vi "Dashboard Main.vi"() -> ()   [LabVIEW 2015]
uses:
  Robot Code/Autonomous Mode.ctl
  <vilib>/Utility/miscctls.llb/LVPointTypeDef.ctl
  <vilib>/Utility/miscctls.llb/LVPositionTypeDef.ctl
  <vilib>/Utility/miscctls.llb/LVRectTypeDef.ctl
  <vilib>/Utility/miscctls.llb/LVRowAndColumnTypeDef.ctl
  <vilib>/event_ctls.llb/eventvkey.ctl
  Operator-Interface-Control-Board.git/trunk/LabVIEW/PWM_Output_TypeDef.ctl
  Operator-Interface-Control-Board.git/trunk/LabVIEW/LED_Output_TypeDef.ctl
  <vilib>/Rock Robotics/Network Tables/NT Read Numeric Array.vi
  <vilib>/Rock Robotics/Network Tables/NT Read Boolean Array.vi
  <vilib>/Rock Robotics/Network Tables/NT Write Boolean Array.vi
  <vilib>/Rock Robotics/Network Tables/NT Write Numeric Array.vi
  <vilib>/Rock Robotics/Network Tables/NT Read Boolean.vi
  <vilib>/Rock Robotics/WPI/Dashboard/WPI_DashboardLogging Global.vi
  <vilib>/vision/driver/NI_Vision_Acquisition_Software.lvlib
panel:
  in  "TCP":refnum<k5>
  out "Image Message":string="Timeout in Camera Communications"
  in  "Dashboard Tab":T1(tab)
  out "Right Drive Speed":dbl(knob) scale=20.0..-20.0
  out "Left Drive Speed":dbl(knob) scale=-20.0..20.0
  out "Robot Direction":dbl(knob) scale=0.0..360.0
  out "Arm Lock State":bool
  out "Distance":string
  out "Front Distance":dbl(slide) scale=0.0..25.0 scale format="%#_g ft"
  out "Arm Mode":string="Disconnected"
  out "Arm Information":cluster{dbl, dbl}(knob)={90.0, 90.0} scale=90.0..220.0 scale format="%d°"
  out "Autonomous Selection":T2
  out "Air Presure":dbl(slide) scale=0.0..150.0 scale format="%#_1f"
  out "Control Board Connection":bool
  out "Network Table Connection":bool
  out "MotorChart R":cluster{"Numeric":dbl, "Numeric":dbl}(graph)
  out "MotorChart L":T3(graph)
  out "MotorSliders R":cluster{"MotorSlide1":dbl, "MotorSlide2":dbl} {"MotorSlide2" scale=-1.0..1.0 scale format="%#_2e"; "MotorSlide1" scale=-1.0..1.0 scale format="%#_2e"}
  out "MotorSliders L":T4 {"MotorSlide4 2" scale=0.0..14.0 scale format="%#_2e"; "MotorSlide2" scale=-1.0..1.0 scale format="%#_2e"; "MotorSlide1" scale=-1.0..1.0 scale format="%#_2e"}
  out "JS1 Z":dbl(slide) scale=-1.0..1.0 scale format="%#_2e"
  out "JS1 Graph":cluster{"X":dbl, "Y":dbl}[](graph)
  out "JS1 Buttons":T5
  out "JS2 Z":dbl(slide) scale=-1.0..1.0 scale format="%#_2e"
  out "JS2 Graph":cluster{"X":dbl, "Y":dbl}[](graph)
  out "JS2 Buttons":T5
  out "Mode":T6(ring)=enum."Auto Disabled"
  in  "DB Camera Config":bool
  out "fps":dbl format="%#.1g"
  out "Mbps":dbl format="%#.1g"
  out "Mbps LED":bool
  in  "Test Slider":dbl(slide) scale=0.0..100.0 scale format="%#_3g"
  in  "On/Off":bool caption="Solenoid"
  in  "Test Name":u16(ring) items=["Select the test to run..."]
  in  "Test Tree":string(tree)
  in  "Motor":cluster{"Value":dbl, "Enable":bool} {"Value" scale=-1.0..1.0 scale format="%#_3g"}
  out "Progress":T7 {"Test Progress" scale=0.0..100.0}
  in  "Rev/Fwd":cluster{"Forward":bool, "Reverse":bool}
  in  "Test Ring":u16(ring) items=["Monochrome", "Color"]
  out "Cmd Status":string
  in  "Execute Command":bool
  in  "Command Params":string[][](table)
  in  "Command Selection":i32(listbox)
  in  "CheckList":i32(listbox)
  out "Tree":string(tree)
  out "Camera Image":T8(plugin-control)
  # "Current"
  # "Set"
  # "Left"
  # "Front"
  # "Right"
  # "Battery"
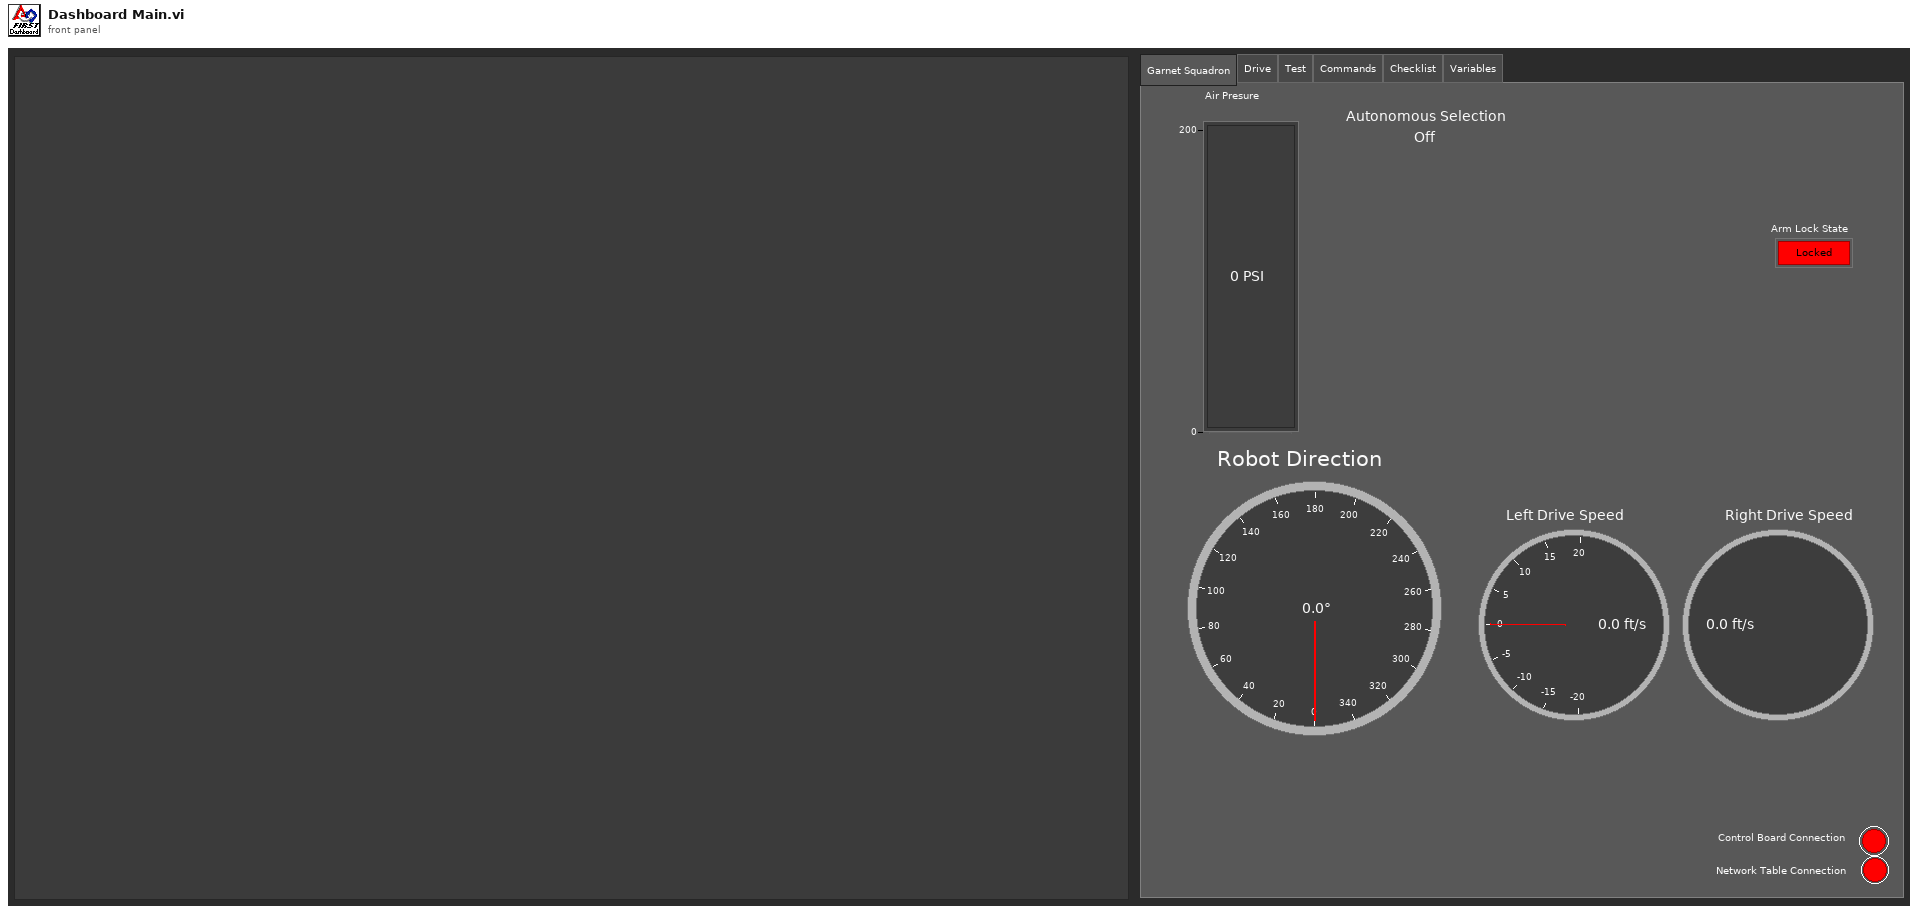
[diagram p1: front panel]
types:
  T1 = enum32{"Garnet Squadron", "Drive", "Test", "Commands", "Checklist", "Variables"}
  T2 = typedef "Autonomous Mode.ctl" = enum16{"Off", "Cross Defense", "Shoot A/B", "Shoot C/D", "Shoot E"}
  T3 = cluster{"Numeric":dbl, "Numeric":dbl, "Battery V":dbl}
  T4 = cluster{"MotorSlide1":dbl, "MotorSlide2":dbl, "MotorSlide4 2":dbl}
  T5 = cluster{bool, bool, bool, bool, bool, bool, bool, bool, bool, bool, bool, bool}
  T6 = enum8{"Tele-Op Disabled", "Tele-Op Enabled", "Auto Disabled", "Auto Enabled", "Test Disabled", "Test Enabled", "Disconnected", "No Code", "E-Stop"}
  T7 = cluster{"Test Progress":u8, "Test Progress Text":string}
  T8 = typedef "IMAQ Image.ctl" = refnum<image>
  T9 = enum32{"Invalid", "Default", "Floating", "Floating/Auto-Hide", "Modal"}
  T10 = typedef "LVRectTypeDef.ctl" = cluster{"Left":i16, "Top":i16, "Right":i16, "Bottom":i16}
  T11 = typedef "LVPositionTypeDef.ctl" = cluster{"Left":i32, "Top":i32}
  T12 = typedef "LVPointTypeDef.ctl" = cluster{"Horizontal":i16, "Vertical":i16}
  T13 = cluster{"IDs":cluster{"RPC field ID":u16, "Unique ID":u16}, "String":string}
  T14 = enum32{"Drive", "Basic", "Custom", "Test", "Checklist", "Variables"}
  T15 = typedef "Image Type" = u32
  T16 = cluster{"Desired Font (Application)":enum16{"User-specified Font", "Application Font", "System Font", "Dialog Font"}, "[User-specified Font]":cluster{"Font Name":string, "Size":i16, "Strikeout?":bool, "Italic?":bool, "Underline?":bool, "Outline?":bool, "Shadow?":bool, "Bold?":bool, "Rotation Angle":dbl}, "Horizontal Alignment":i16, "Vertical Alignment":i16}
  T17 = cluster{"Left":i32, "Top":i32, "Right":i32, "Bottom":i32}
  T18 = typedef "GRIP Contours Report.ctl" = cluster{"area":dbl, "centerX":dbl, "centerY":dbl, "width":dbl, "height":dbl, "solidity":dbl}
  T19 = cluster{"Type":u32, "Version":u32, "Flags":u32, "SerialNumberHigh":u32, "SerialNumberLow":u32, "BusType":u32, "InterfaceName":string, "VendorName":string, "ModelName":string, "CameraFileName":string, "CameraAttributeURL":string}[]
  T20 = cluster{"Type":u32, "Version":u32, "Flags":u32, "SerialNumberHigh":u32, "SerialNumberLow":u32, "BusType":u32, "InterfaceName":string, "VendorName":string, "ModelName":string, "CameraFileName":string, "CameraAttributeURL":string}
  T21 = typedef "IMAQdx.ctl" = refnum<k21>
  T22 = typedef "NI_LVConfig.lvlib/Config Data RefNum.ctl" = refnum<k1>
  T23 = typedef "LED_Output_TypeDef.ctl" = cluster{"LED 0":bool, "LED 1":bool, "LED 2":bool, "LED 3":bool, "LED 4":bool, "LED 5":bool, "LED 6":bool, "LED 7":bool, "LED 8":bool, "LED 9":bool, "LED 10":bool, "LED 11":bool, "LED 12":bool, "LED 13":bool, "LED 14":bool, "LED 15":bool}
  T24 = typedef "PWM_Output_TypeDef.ctl" = cluster{"PWM 0":u8, "PWM 1":u8, "PWM 2":u8, "PWM 3":u8, "PWM 4":u8, "PWM 5":u8, "PWM 6":u8, "PWM 7":u8, "PWM 8":u8, "PWM 9":u8, "PWM 10":u8}
  T25 = typedef "Analog_Input_TypeDef.ctl" = cluster{"ANA 0":u8, "ANA 1":u8, "ANA 2":u8, "ANA 3":u8, "ANA 4":u8, "ANA 5":u8, "ANA 6":u8, "ANA 7":u8, "ANA 8":u8, "ANA 9":u8, "ANA 10":u8, "ANA 11":u8, "ANA 12":u8, "ANA 13":u8, "ANA 14":u8, "ANA 15":u8}
  T26 = typedef "Switch_Input_TypeDef.ctl" = cluster{"SW 0":bool, "SW 1":bool, "SW 2":bool, "SW 3":bool, "SW 4":bool, "SW 5":bool, "SW 6":bool, "SW 7":bool, "SW 8":bool, "SW 9":bool, "SW 10":bool, "SW 11":bool, "SW 12":bool, "SW 13":bool, "SW 14":bool, "SW 15":bool}
  T27 = cluster{"Error Strings":string, "Disable Counts":cluster{u16, u16}, "Rail Faults":cluster{u16, u16, u16}, "Robot IP":string, "DB Mode":u8, "Event Info":cluster{"Name":string, "Type":u8, "Number":u16, "Replay":u8}, "Camera Addr":string}
  T28 = cluster{"Storage":cluster{"Disk Free":u64, "RAM Block":u32, "RAM free":u32}, "CPU Utilization":cluster{"CPU % ISR":sgl, "CPU % Time Crit":sgl, "CPU % Timed Str":sgl, "CPU % High":sgl, "CPU % Above":sgl, "CPU % Normal":sgl, "CPU % Low":sgl}, "CAN":cluster{"% Bus Utilization":sgl, "Bus Off Cnt":u32, "TX_FIFO Full Cnt":u32, "Receive Error Cnt":u8, "Transmit Error Cnt":u8}, "HID":cluster{"HID Outputs":u32, "Rumble Low":u16, "Rumble High":u16}[]}
  T29 = cluster{"Status bits":cluster{"Test Mode":bool, "Autonomous":bool, "Enabled":bool, "Code Start":bool, "Brownout":bool, "Reserved 2":bool, "Reserved 3":bool, "E-Stop":bool}, "Code Trace":cluster{"Disabled":bool, "TeleOp":bool, "Auto":bool, "Test":bool}, "Controller Type":enum16{"unknown", "cRIO", "roboRio"}, "Code?":enum16{"unknown", "noCode", "code"}, "Battery V":dbl}
  T30 = cluster{"Control Bits":cluster{"TestMode":bool, "Autonomous":bool, "Enabled":bool, "FMS Present":bool, bool, bool, bool, "E-Stop":bool}, "Team Station ":u8, "Countdown":sgl, "Joystick Values":cluster{"Axes":dbl[], "Buttons":bool[], "POVs":i16[]}[]}
  T31 = cluster{"Axes":dbl[], "Buttons":bool[], "POVs":i16[]}[]
  T32 = cluster{"Axes":dbl[], "Buttons":bool[], "POVs":i16[]}
  T33 = cluster{"Buttons[0]":bool, "Buttons[1]":bool, "Buttons[2]":bool, "Buttons[3]":bool, "Buttons[4]":bool, "Buttons[5]":bool, "Buttons[6]":bool, "Buttons[7]":bool, "Buttons[8]":bool, "Buttons[9]":bool, "Buttons[10]":bool, "Buttons[11]":bool}
  T34 = cluster{"Operation":enum16{"Update", "Clear"}, "Color Box":u32}[]
  T35 = typedef "eventvkey.ctl" = enum16{"ASCII", "Enter", "Return", "Shift", "Ctrl", "Alt", "Cmd", "Opt", "Caps", "NumLock", "Clear", "Break", "Up", "Down", "Left", "Right", "Insert", "Delete", "Home", "End", "PageUp", "PageDown", "Escape", "Help", "Pause", "ScrollLock", "F1", "F2", "F3", "F4", "F5", "F6", "F7", "F8", "F9", "F10", "F11", "F12", "F13", "F14", "F15", "F16", "F17", "F18", "F19", "F20", "F21", "F22", "F23", "F24", "Play", "VolumeUp", "VolumeDown", "Mute", "Two Byte Char"}
  T36 = cluster{"Operation":enum16{"Update", "Clear"}, "Color Box":u32}
  T37 = typedef "LVRowAndColumnTypeDef.ctl" = cluster{"Row":i32, "Column":i32}
  T38 = cluster{"Shift":bool, "Ctrl":bool, "Alt":bool, "Cmd":bool, "Opt":bool}
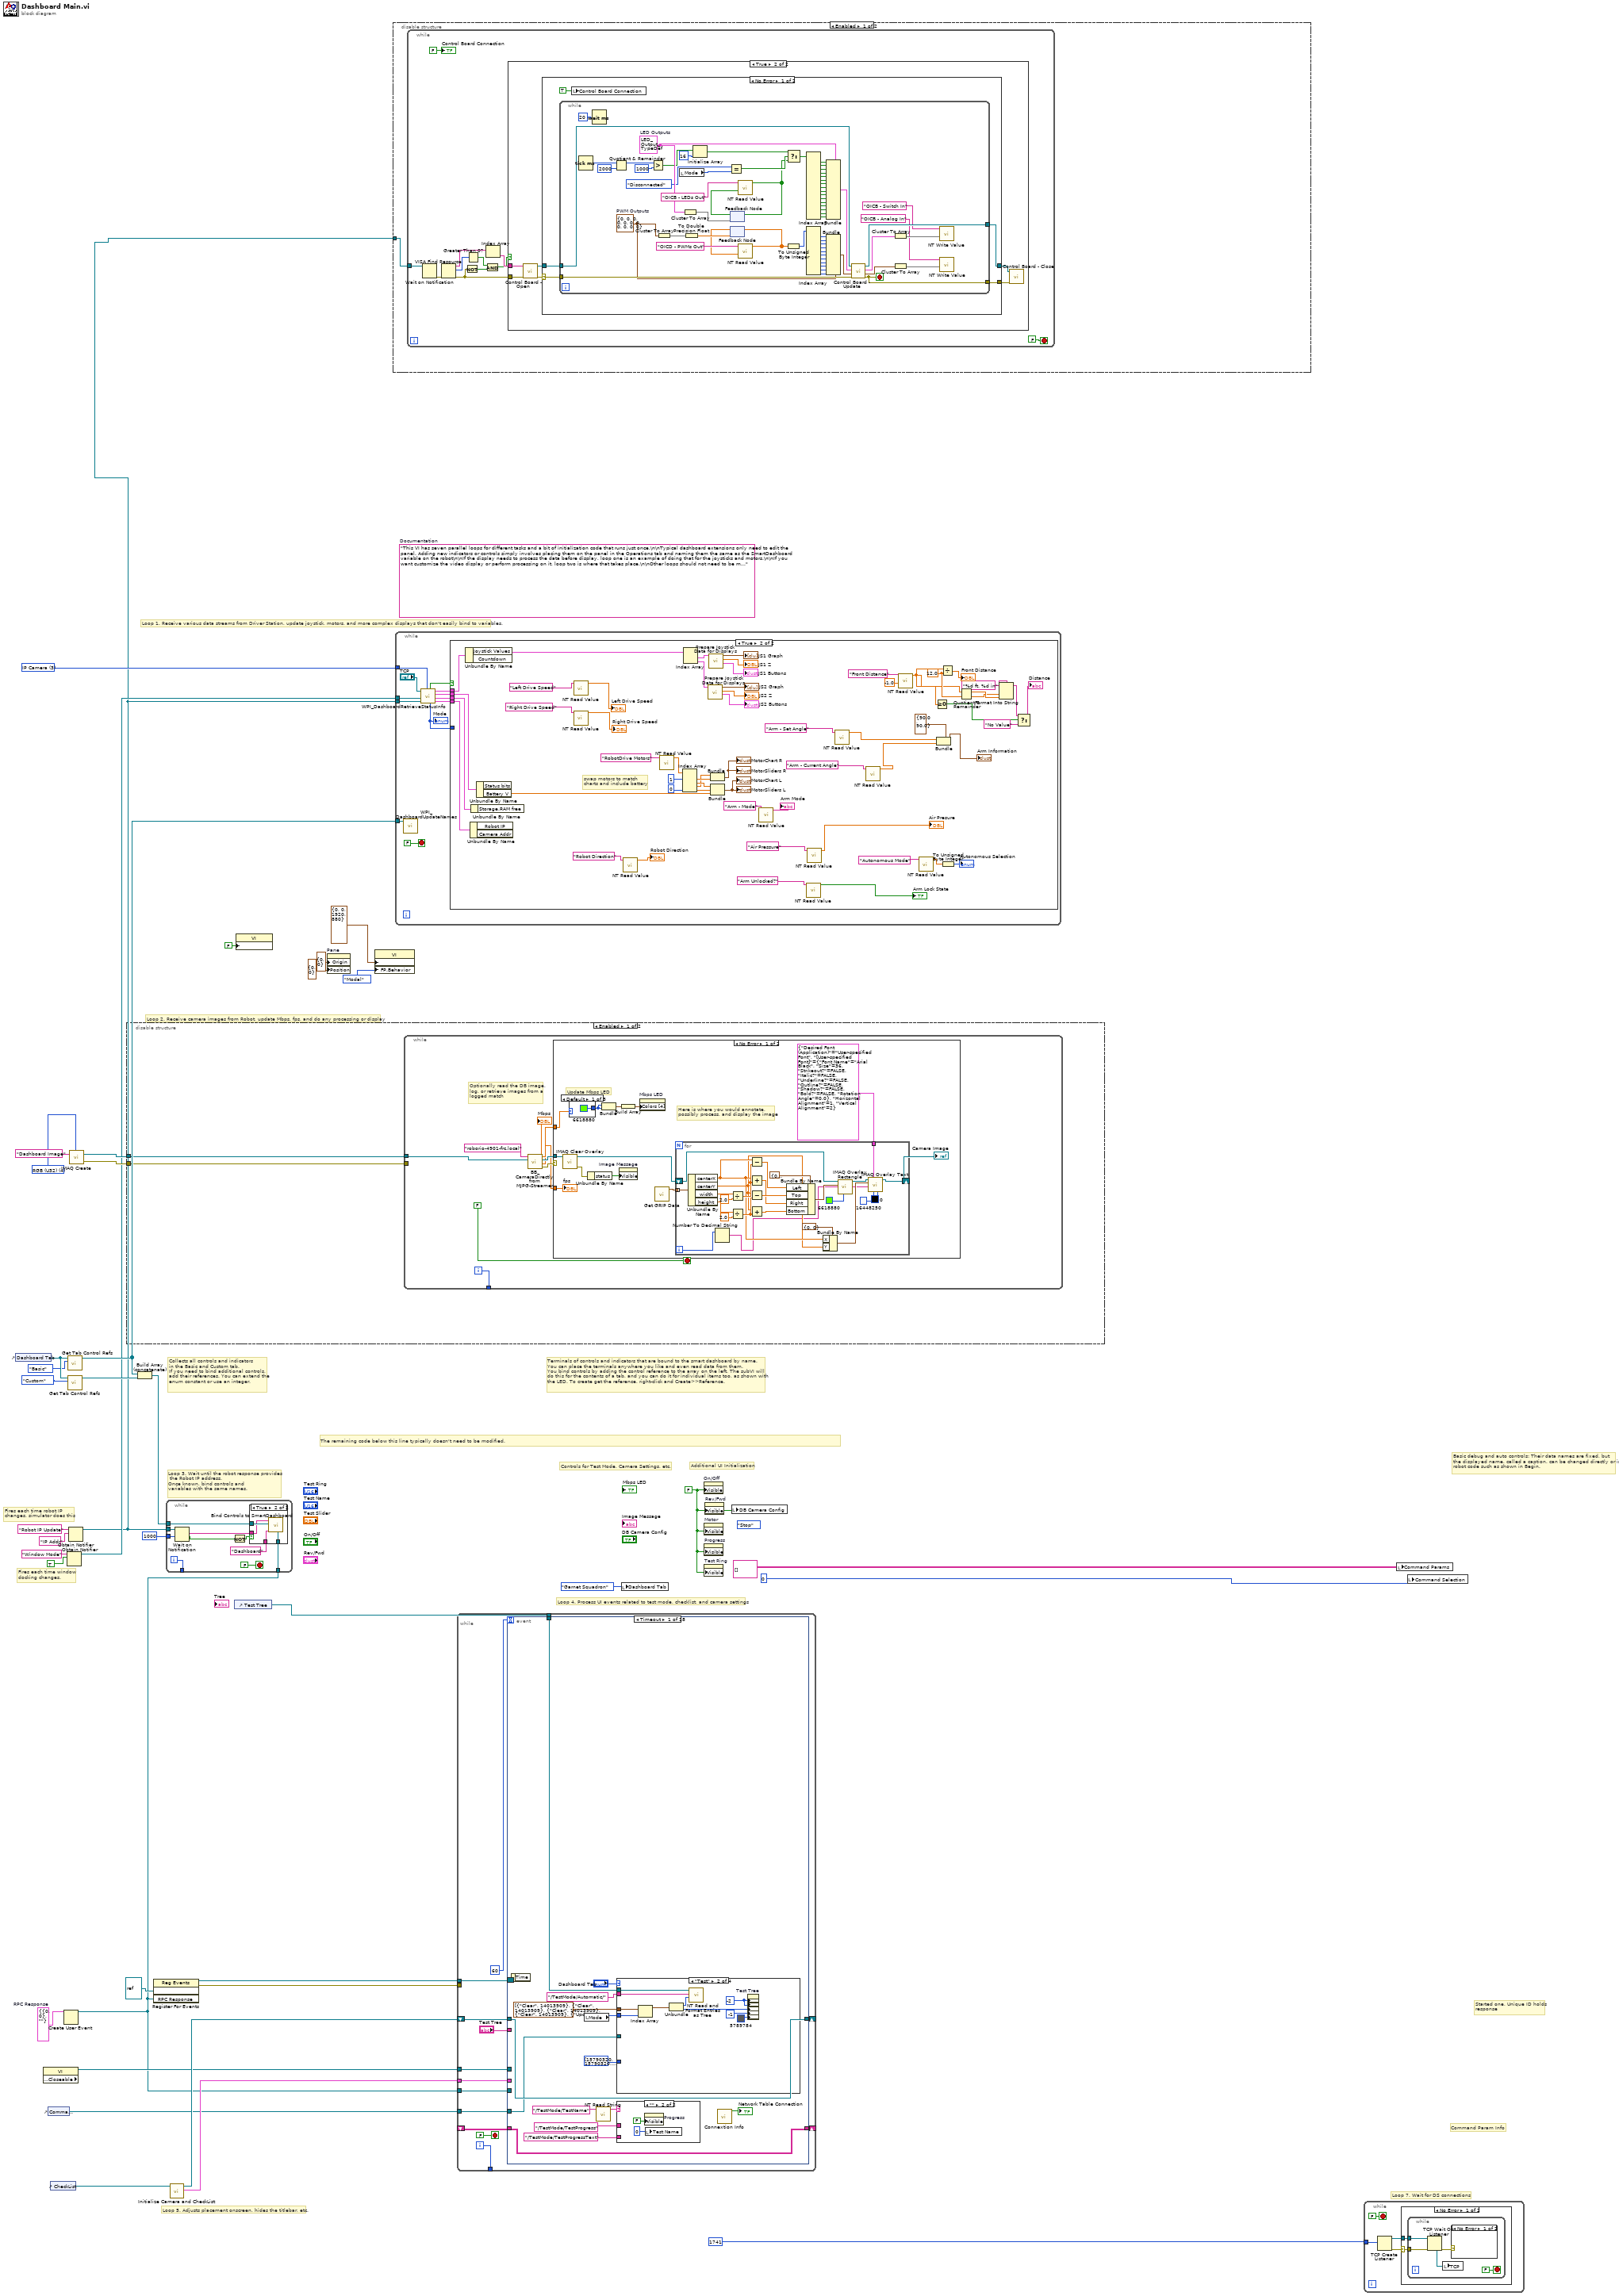
[diagram p0: block diagram]
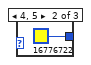
[diagram p2: hidden frame]
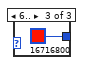
[diagram p3: hidden frame]
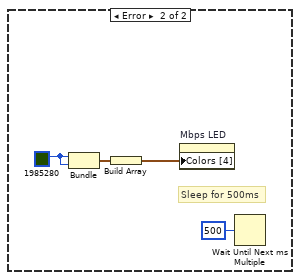
[diagram p4: hidden frame]
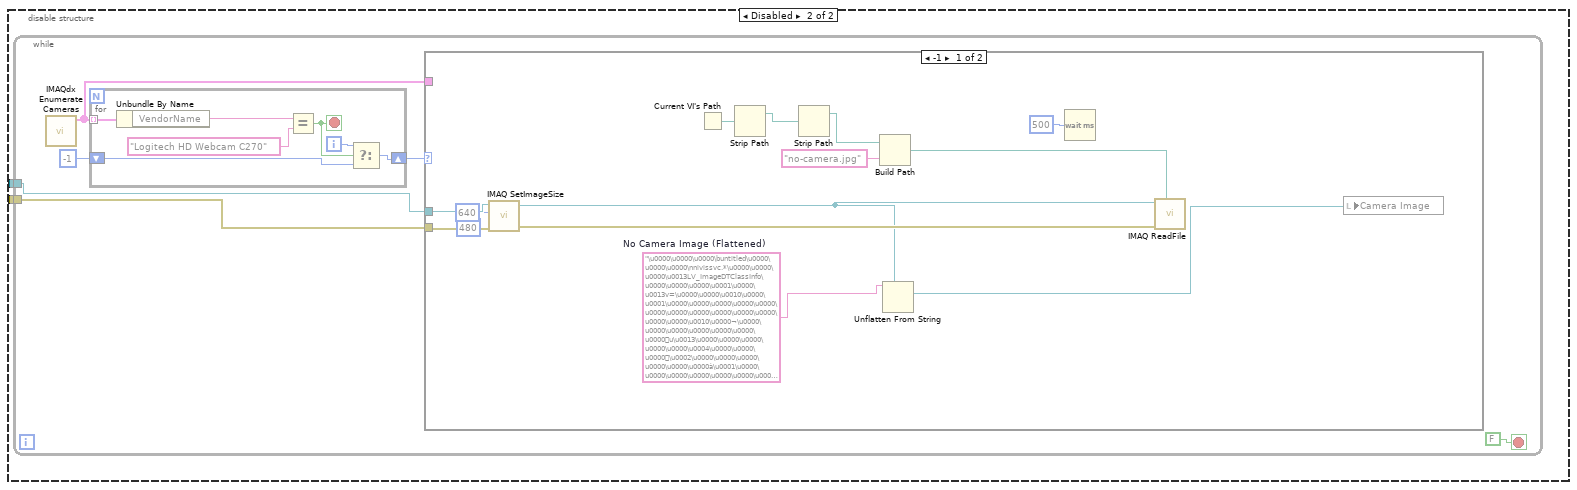
[diagram p5: hidden frame]
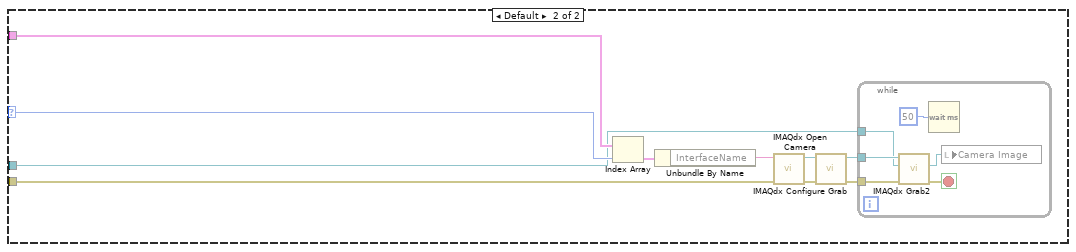
[diagram p6: hidden frame]
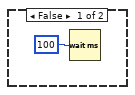
[diagram p7: hidden frame]
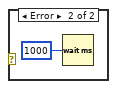
[diagram p10: hidden frame]
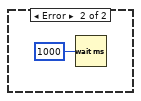
[diagram p11: hidden frame]
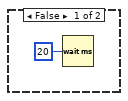
[diagram p12: hidden frame]
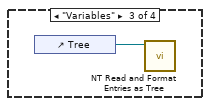
[diagram p15: hidden frame]
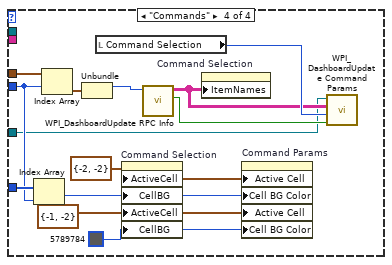
[diagram p16: hidden frame]
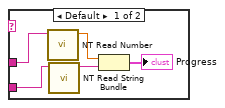
[diagram p17: hidden frame]
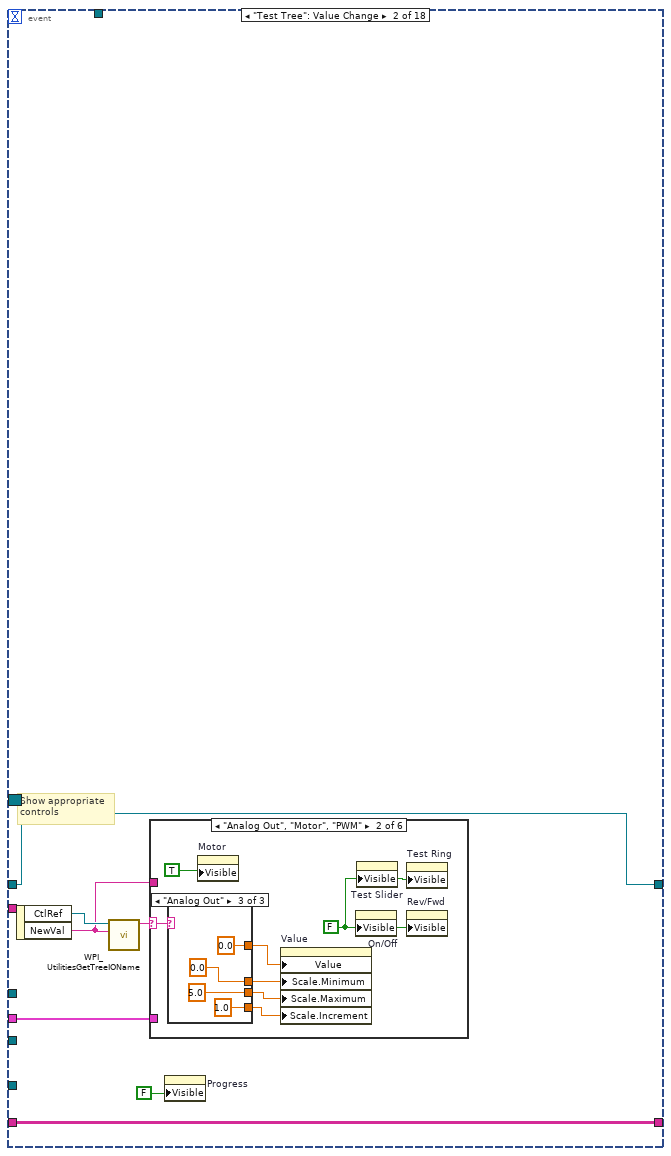
[diagram p18: hidden frame]
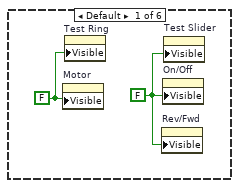
[diagram p19: hidden frame]
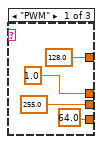
[diagram p20: hidden frame]
diagram:
  w7 = u16 3 items=["Camera Off", "USB Camera SW", "USB Camera HW", "IP Camera"] ("Vision")
  w12 = T13 {"IDs"={"RPC field ID"=0, "Unique ID"=0}, "String"=""}  # RPC Response
  (unwired) enum32{"Stop", "Record", "Playback"}."Stop" ("Rec Mode")
  w17 = FALSE ("Visible")
  (unwired) "This VI has seven parallel loops for different tasks and a bit of initialization code that runs just once.\n\nTypical dashboard extensions only need to edit the panel. Adding new indicators or controls simply involves placing them on the panel in the Operations tab and naming them the same as the SmartDashboard variable on the robot\n\nIf the display needs to process the data before display, loop one is an example of doing that for the joysticks and motors.\n\nIf you want customize the video display or perform processing on it, loop two is where that takes place.\n\nOther loops should not need to be modified. They are pretty standard, and document the task they perform."  # Documentation
  w39 = T15 4 items=["Grayscale (U8)", "Grayscale (I16)", "Grayscale (SGL)", "Complex (CSG)", "RGB (U32)", "HSL (U32)", "RGB (U64)"] ("Image Type")
  # "Command Param Info"
  # "Started one, Unique ID holds\nresponse"
  # "Loop 7. Wait for DS connections"
  # "Basic debug and auto controls: Their data names are fixed, but\nthe displayed name, called a caption, can be changed directly or in\nrobot code such as shown in Begin."
  # "Controls for Test Mode, Camera Settings, etc."
  # "Additional UI Initialization"
  # "Fires each time robot IP\nchanges, simulator does this"
  # "Fires each time window\ndocking changes."
  # "Collects all controls and indicators\nin the Basic and Custom tab.\nIf you need to bind additional controls,\nadd their references. You can extend the\nenum constant or use an integer."
  # "The remaining code below this line typically doesn't need to be modified."
  # "Loop 4. Process UI events related to test mode, checklist, and camera settings"
  # "Terminals of controls and indicators that are bound to the smart dashboard by name.\nYou can place the terminals anywhere you like and even read data from them.\nYou bind controls by adding the control reference to the array on the left. The subVI will\ndo this for the contents of a tab, and you can do it for individual items too, as shown with\nthe LED. To create get the reference, right-click and Create>>Reference."
  # "Loop 3. Wait until the robot response provides\n the Robot IP address.\nOnce known, bind controls and\nvariables with the same names."
  # "Loop 5. Adjusts placement onscreen, hides the titlebar, etc."
  # "Loop 1. Receive various data streams from Driver Station, update joystick, motors, and more complex displays that don't easily bind to variables."
  # "Loop 2. Receive camera images from Robot, update Mbps, fps, and do any processing or display"
  n1 = control-ref of="Dashboard Tab"() -> (w23:refnum<vi>)
  n2 = property class="VI" props=["Front Panel.Closeable"]() -> (reference out=w24:refnum<vi>)  [unwired: 2 in, 2 out]
  n3 = control-ref of="Command Params"() -> (w8:refnum<vi>)
  n4 = control-ref of="CheckList"() -> (w18:refnum<vi>)
  n5 = Create User Event(user event datatype=w12) -> (user event=w9:refnum<user-event>)  [unwired: 1 in, 1 out]
  n6 = Obtain Notifier(name (unnamed)="Window Mode", notification data type=TRUE) -> (notifier out=w15:refnum<notifier>)  [unwired: 2 in, 2 out]
  n7 = call <vilib>:"Get Tab Control Refs.vi"("Page Index"=T14."Basic" ("Dashboard Tab"), "TabControl in"=w23) -> ("ControlsOnPage"=w16:refnum<vi>[])  [unwired: 9 in]
  n8 = call <vilib>:"Get Tab Control Refs.vi"("Page Index"=T14."Custom" ("Dashboard Tab"), "TabControl in"=w23) -> ("ControlsOnPage"=w22:refnum<vi>[])  [unwired: 9 in]
  n9 = Obtain Notifier(name (unnamed)="Robot IP Update", notification data type="IP Addr" ("name (unnamed)")) -> (notifier out=w6:refnum<notifier>)  [unwired: 2 in, 2 out]
  n10 = call "IMAQ Create"("Image Name"="Dashboard Image", "Image Type"=w39) -> ("New Image"=w37:T8, "error out"=w36:errorcluster)  [unwired: 2 in, 1 out]
  n11 = disable-structure shown="Enabled" {
    disable-tunnel: w37 -> [w41 w96]
    disable-tunnel: w36 -> [w40 w95]
    frame Enabled {
      n12 = while {
        tunnel: w41 -> [w47]
        tunnel: w40 -> [_]
        tunnel: [w48] -> _
        i -> [w48]
        stop <- FALSE stop-if-true
        # "Optionally read the DB image,\nlog, or retrieve images from a\nlogged match"
        n13 = call "BB_CameraDirectly from MJPG-Streamer.vi"("Image"=w47, "address"="roborio-4901-frc.local" ("Camera IP")) -> ("error out"=w45:errorcluster, "Bandwidth (Mbps)"=w43:dbl, "Image Out"=w46:T8, "FPS"=w44:dbl)  [unwired: 6 in]
        "Mbps" <- w43
        n14 = case shown="No Error" w45 {
          tunnel: w46 -> [w56 _]
          tunnel: w43 -> [w55 _]
          tunnel: w44 -> [w54 _]
          frame No Error {
            # "Here is where you would annotate,\npossibly process, and display the image"
            # "Update Mbps LED"
            n15 = call "IMAQ Clear Overlay"("Image"=w56) -> ("error out"=w60:errorcluster, "Image Out"=w53:T8)  [unwired: 2 in, 7 out]
            n16 = case shown="Default" w55 {
              tunnel: [u32 6618880 ("Color Box") u32 16776722 ("Color Box") u32 16716800 ("Color Box")] -> w57
              frame Default {
              }
              frame 4, 5 {
              }
              frame 6.. {
              }
            }
            n17 = Unbundle By Name(w60) -> ("status"=w61:bool)
            n18 = Bundle("Color Box"=w57, "Color Box"=w57) -> (w59:cluster{"Color Box":u32, "Color Box":u32})  [unwired: 1 out]
            n19 = property on="Image Message" class="Str"("Visible"=w61) -> ()  [unwired: 2 in, 2 out]
            n20 = Build Array(w59) -> (w58:cluster{"Color Box":u32, "Color Box":u32}[])
            n21 = property on="Mbps LED" class="Bool (strict)"("Colors [4]"=w58) -> ()  [unwired: 2 in, 2 out]
            n22 = call "Get GRIP Data.vi"() -> ("ContoursReport"=w51:T18[])  [unwired: 9 in, 2 out]
            n23 = for {
              shift-right: [w65] -> w52
              shift-left: w53 -> [w87]
              tunnel: w51 -> [w85] mode=indexing
              tunnel: T16 {"Desired Font (Application)"=enum."User-specified Font", "[User-specified Font]"={"Font Name"="Arial Black", "Size"=36, "Strikeout?"=FALSE, "Italic?"=FALSE, "Underline?"=FALSE, "Outline?"=FALSE, "Shadow?"=FALSE, "Bold?"=FALSE, "Rotation Angle"=0.0}, "Horizontal Alignment"=1, "Vertical Alignment"=2} ("Font, Size & Style") -> [w64]
              i -> [w68]
              n24 = Unbundle By Name(w85) -> ("centerX"=w72:dbl, "centerY"=w70:dbl, "width"=w83:dbl, "height"=w80:dbl)
              n25 = Number To Decimal String(number=w68) -> (decimal integer string=w67:string)  [unwired: 1 in]
              n26 = Divide(x=w83, y=2.0) -> (x/y=w78:dbl)
              n27 = Divide(x=w80, y=2.0) -> (x/y=w79:dbl)
              n28 = Subtract(x=w72, y=w78) -> (x-y=w75:dbl)
              n29 = Add(x=w72, y=w78) -> (x+y=w71:dbl)
              n30 = Subtract(x=w70, y=w79) -> (x-y=w74:dbl)
              n31 = Add(x=w70, y=w79) -> (x+y=w73:dbl)
              n32 = Bundle By Name(cluster=T17 {"Left"=0, "Top"=0, "Right"=0, "Bottom"=0} ("Rectangle"), "Left"=w75, "Top"=w74, "Right"=w71, "Bottom"=w73) -> (w76:T17)
              n33 = Bundle By Name(cluster=cluster{"X":i32, "Y":i32} {"X"=0, "Y"=0} ("Point"), "X"=w72, "Y"=w70) -> (w69:cluster{"X":i32, "Y":i32})
              n34 = call "IMAQ Overlay Rectangle"("Color"=u32 6618880, "Rectangle"=w76, "Image"=w87) -> ("Image Out"=w66:T8)  [unwired: 7 in, 1 out]
              n35 = call "IMAQ Overlay Text"("BG Color (Transparent)"=u32 0, "Text Color (black)"=u32 16448250, "Font, Size & Style"=w64, "String"=w67, "Origin"=w69, "Image"=w66) -> ("Image Out"=w65:T8)  [unwired: 4 in, 1 out]
            }
            "Camera Image" <- w52
            "fps" <- w54
          }
          frame Error {
            w92 = u32 1985280 ("Color Box")
            # "Sleep for 500ms"
            n36 = Bundle("Color Box"=w92, "Color Box"=w92) -> (w94:cluster{"Color Box":u32, "Color Box":u32})  [unwired: 1 out]
            n37 = Build Array(w94) -> (w93:cluster{"Color Box":u32, "Color Box":u32}[])
            n38 = property on="Mbps LED" class="Bool (strict)"("Colors [4]"=w93) -> ()  [unwired: 2 in, 2 out]
            n39 = Wait Until Next ms Multiple(millisecond multiple=u32 500) -> ()  [unwired: 1 out]
          }
        }
      }
    }
    frame Disabled {
      n40 = while {
        tunnel: w96 -> [w98]
        tunnel: w95 -> [w97]
        stop <- FALSE stop-if-true
        n41 = call <vilib>:"IMAQdx Enumerate Cameras.vi"() -> ("Camera Information Array"=w100:T19)  [unwired: 10 in, 1 out]
        n42 = for {
          tunnel: w100 -> [w139] mode=indexing
          shift-right: [w133] -> w101
          shift-left: -1 -> [w135]
          i -> [w136]
          stop <- w134 stop-if-true
          n43 = Unbundle By Name(w139) -> ("VendorName"=w138:string)
          n44 = Equal?(x=w138, y="Logitech HD Webcam C270") -> (x = y?=w134:bool)
          n45 = Select(t=w136, s=w134, f=w135) -> (s? t:f=w133:i32)
        }
        n46 = case shown="-1" w101 {
          selector: w101 -> [_ w123]
          tunnel: w98 -> [w113 w119]
          tunnel: w97 -> [w112 w118]
          tunnel: w100 -> [_ w124]
          frame -1 {
            w103 = "\u0000\u0000\u0000\buntitled\u0000\u0000\u0000\nnivissvc.*\u0000\u0000\u0000\u0013LV_ImageDTClassInfo\u0000\u0000\u0000\u0001\u0000\u0013v=\u0000\u0000\u0010\u0000\u0001\u0000\u0000\u0000\u0000\u0000\u0000\u0000\u0000\u0000\u0000\u0000\u0000\u0000\u0010\u0000¬\u0000\u0000\u0000\u0000\u0000\u0000\u0000u\u0013\u0000\u0000\u0000\u0000\u0000\u0004\u0000\u0000\u0000\u0002\u0000\u0000\u0000\u0000\u0000\u0000à\u0001\u0000\u0000\u0000\u0000\u0000\u0000\u0003\u0000\u0000\u0000\u0000\u0000\u0000\u0000\u0000\u0000\u0000\u0000\u0000\u0000\u0000\u0000\u0000\u0000\u0000\u0000\u0000\u0000\u0000\u0000\u0000\u0000\u0000\u0000\u0002\u0000\u0000\u0000\u0000\u0000\u0000\u0000\u0000\u0000\u0000\u0010\u0003E\n\u0000\u0000\u0000\u0000,ºc\u000f\u0000\u0000\u0000\u0000\u0000\u0005<z\u0000\u0000\u0000\b<\u0000\u0000\u0000\u0000\u0000\u0000\u0000\u0000\u0000\u0000\u0001\u0000\u0000\u0000\u0001\u0000\u0000\u0000\u0000\u0000\u0000\u0000\b\u0000\u0000\u0000u\u0013\u0000\u0000\u0000\u0000\u0000\u0000\u0000\u0000\u0000\u0000\u0000\u0000\u0000\t\u0000\u0000\u0000\u0000\u0000\u0000\u0000untitled\u0000\u0000\u0000\u0000\u0000\u0000\u0000\u0000\u0000\u0000\u0000\u0000\u0000\u0000\u0000\u0000\u0000\u0000\u0000\u0000\u0000\u0000\u0000\u0000\u0000\u0000\u0000\u0000\u0000\u0000\u0000\u0000\u0000\u0000\u0000\u0000\u0000\u0000\u0000\u0000\u0000\u0000\u0000\u0000\u0000\u0000\u0000\u0000\u0000\u0000\u0000\u0000\u0000\u0000\u0000\u0000\u0000\u0000\u0000\u0000\u0000\u0000\u0000\u0000\u0000\u0000\u0000\u0000\u0000\u0000\u0000\u0000\u0000\u0000\u0000\u0000\u0000\u0000\u0000\u0000\u0000\u0000\u0000\u0000\u0000\u0000\u0000\u0000\u0000\u0000\u0000\u0000\u0000\u0000\u0000\u0000\u0000\u0000\u0000\u0000\u0000\u0000\u0000\u0000\u0000\u0000\u0000\u0000\u0000\u0000\u0000\u0000\u0000\u0000\u0000\u0000\u0000\u0000\u0000\u0000\u0000\u0000\u0000\u0000\u0000\u0000\u0000\u0000\u0000\u0000\u0000\u0000\u0000\u0000\u0000\u0000\u0000\u0000\u0000\u0000\u0000\u0000\u0000\u0000\u0000\u0000\u0000\u0000\u0000\u0000\u0000\u0000\u0000\u0000\u0000\u0000\u0000\u0000\u0000\u0000\u0000\u0000\u0000\u0000\u0000\u0000\u0000\u0000\u0000\u0000\u0000\u0000\u0000\u0000\u0000\u0000\u0000\u0000\u0000\u0000\u0000\u0000\u0000\u0000\u0000\u0000\u0000\u0000\u0000\u0000\u0000\u0000\u0000\u0000\u0000\u0000\u0000\u0000\u0000\u0000\u0000\u0000\u0000\u0000\u0000\u0000\u0000\u0000\u0000\u0000\u0000\u0000\u0000\u0000\u0000\u0000\u0000\u0000\u0000\u0000\u0000\u0000\u0000\u0000\u0000\u0000\u0000\u0000\u0000\u0000\u0000\u0000\u0000\u0000\u0000\u0000\u0000\u0000\u0000\u0000\u0000\u0000\u0000\u0000\u0000\u0000\u0000\u0000\u0000\u0000\u0000\u0000\u0000\u0000\u0000\u0000\u0000\u0000\u0000\u0000\u0000\u0000\u0000\u0000\u0000\u0000\u0000\u0000\u0000\u0000\u0000\u0000\u0000\u0000\u0000\u0000\u0000\u0000\u0000\u0000\u0000\u0000\u0000\u0000\u0000\u0000\u0000\u0000\u0000\u0000\u0000\u0000\u0000\u0000\u0000\u0000\u0000\u0000\u0000\u0000\u0000\u0000\u0000\u0000\u0000\u0000\u0000\u0000\u0000\u0000\u0000\u0000\u0000\u0000\u0000\u0000\u0000\u0000\u0000\u0000\u0000\u0000\u0000\u0000\u0000\u0000\u0000\u0000\u0000\u0000\u0000\u0000\u0000\u0000\u0000\u0000\u0000\u0000\u0000\u0000\u0000\u0000\u0000\u0000\u0000\u0000\u0000\u0000\u0000\u0000\u0000\u0000\u0000\u0000\u0000\u0000\u0000\u0000\u0000\u0000\u0000\u0000\u0000..."  # No Camera Image (Flattened)
            n47 = call "IMAQ SetImageSize"("error in (no error)"=w112, "Y Resolution"=480, "X Resolution"=640, "Image"=w113) -> ("error out"=w109:errorcluster, "Image Out"=w105:T8)  [unwired: 1 in]
            n48 = Current VI's Path() -> (path=w108:path)
            n49 = Strip Path(path=w108) -> (stripped path=w107:path)  [unwired: 1 out]
            n50 = Strip Path(path=w107) -> (stripped path=w106:path)  [unwired: 1 out]
            n51 = Build Path(base path=w106, name or relative path="no-camera.jpg") -> (appended path=w115:path)
            n52 = Unflatten From String(type=w105, binary string=w103) -> (value=w104:T8)  [unwired: 3 in, 2 out]
            n53 = Wait (ms)(milliseconds to wait=u32 500) -> ()  [unwired: 1 out]
            n54 = call "IMAQ ReadFile"("File Path"=w115, "error in (no error)"=w109, "Image"=w105) -> ()  [unwired: 4 in, 5 out]
            n55 = local write "Camera Image"(w104) -> ()
          }
          frame Default {
            n56 = Index Array(array=w124, index=w123) -> (element=w122:T20)
            n57 = Unbundle By Name(w122) -> ("InterfaceName"=w121:string)
            n58 = call <vilib>:"IMAQdx Open Camera.vi"("error in"=w118, "Session In"=w121) -> ("error out"=w126:errorcluster, "Session Out"=w125:T21)  [unwired: 8 in]
            n59 = call <vilib>:"IMAQdx Configure Grab.vi"("error in"=w126, "Session In"=w125) -> ("error out"=w117:errorcluster, "Session Out"=w120:T21)  [unwired: 8 in]
            n60 = while {
              tunnel: w120 -> [w132]
              tunnel: w119 -> [w130]
              tunnel: w117 -> [w131]
              stop <- w129 stop-if-true
              n61 = call <vilib>:"IMAQdx Grab2.vi"("error in"=w131, "Image In"=w130, "Session In"=w132) -> ("error out"=w129:errorcluster, "Image Out"=w127:T8)  [unwired: 5 in, 2 out]
              n62 = Wait (ms)(milliseconds to wait=u32 50) -> ()  [unwired: 1 out]
              n63 = local write "Camera Image"(w127) -> ()
            }
          }
        }
      }
    }
  }
  n64 = Build Array (concatenate)(w16, w22) -> (w21:refnum<vi>[])
  n65 = register-events(refnum<vi> refnum, w9) -> (reference out=w28:refnum<event-registration>, error out=w27:errorcluster)  [unwired: 2 in]
  n66 = while {
    tunnel: w21 -> [w149]
    tunnel: w6 -> [w147]
    tunnel: [w145] -> _
    tunnel: u32 1000 ("milliseconds to wait") -> [w144]
    tunnel: w9 -> [w140]
    i -> [w145]
    stop <- FALSE stop-if-true
    n67 = Wait on Notification(notifier=w147, timeout in ms (-1)=w144) -> (notification=w146:string, timed out?=w142:bool)  [unwired: 2 in, 2 out]
    n68 = Not(x=w142) -> (.not. x?=w143:bool)
    n69 = case shown="True" w143 {
      tunnel: w149 -> [_ w153]
      tunnel: w146 -> [_ w152]
      tunnel: "Dashboard" -> [_ w151]
      tunnel: w140 -> [_ w150]
      frame False {
      }
      frame True {
        n70 = call <vilib>:"Bind Controls to SmartDashboard.vi"("RPC ref"=w150, "Client Name"=w151, "Bound Control Refs"=w153, "Server IP Address"=w152) -> ()  [unwired: 8 in]
      }
    }
  }
  n71 = call "Initialize Camera and CheckList.vi"("ListBox in"=w18) -> ("Array"=w31:cluster{string[]}[], "File Refnum"=w30:T22)  [unwired: 8 in, 1 out]
  n72 = control-ref of="Test Tree"() -> (w29:refnum<vi>)
  n73 = property class="VI"("Front Panel.TitleBarVis"=FALSE ("Front Panel Window:Title Bar Visible")) -> ()  [unwired: 2 in, 2 out]
  n74 = property on="Pane" class="Pane"("Origin"=T12 {"Horizontal"=0, "Vertical"=0}, "Position"=T11 {"Left"=0, "Top"=0}) -> ()  [unwired: 2 in, 2 out]
  n75 = property class="VI"("Front Panel.WinBounds"=T10 {"Left"=0, "Top"=0, "Right"=1920, "Bottom"=880} ("Front Panel Window:Window Bounds"), "FP.Behavior"=T9."Modal" ("Front Panel Window:Behavior")) -> ()  [unwired: 2 in, 2 out]
  n76 = disable-structure shown="Enabled" {
    disable-tunnel: w6 -> [w154 _]
    frame Enabled {
      n77 = while {
        tunnel: w154 -> [w155]
        stop <- FALSE stop-if-true
        n78 = Wait on Notification(notifier=w155) -> (error out=w156:errorcluster)  [unwired: 3 in, 3 out]
        n79 = VISA Find Resource(8:w156) -> (0:w159:errorcluster, 2:w165:u32, 3:w164:string[])  [unwired: 2 in]
        n80 = Not(x=w159) -> (.not. x?=w160:bool)
        n81 = Greater Than 0?(x=w165) -> (x > 0?=w162:bool)
        n82 = And(x=w162, y=w160) -> (x .and. y?=w161:bool)
        n83 = Index Array(array=w164) -> (element=w163:string)  [unwired: 1 in]
        n84 = case shown="True" w161 {
          tunnel: w163 -> [_ w171]
          tunnel: w159 -> [_ w170]
          frame False {
            n85 = Wait (ms)(milliseconds to wait=u32 100) -> ()  [unwired: 1 out]
          }
          frame True {
            n86 = call "Control Board - Open.vi"("error in (no error)"=w170, "VISA Refnum in"=w171) -> ("error out"=w169:errorcluster, "VISA Refnum out"=w172:refnum<visa-resource-name>)  [unwired: 8 in]
            n87 = case shown="No Error" w169 {
              selector: w169 -> [w176 w242]
              tunnel: w172 -> [w177 w241]
              tunnel: [w174 w242] -> w168
              tunnel: [w173 w241] -> w167
              frame No Error {
                n88 = while {
                  tunnel: w177 -> [w240]
                  tunnel: [w239] -> w173
                  tunnel: [w237] -> w174
                  tunnel: w176 -> [w238]
                  stop <- w237 stop-if-true
                  w210 = T23 {"LED 0"=FALSE, "LED 1"=FALSE, "LED 2"=FALSE, "LED 3"=FALSE, "LED 4"=FALSE, "LED 5"=FALSE, "LED 6"=FALSE, "LED 7"=FALSE, "LED 8"=FALSE, "LED 9"=FALSE, "LED 10"=FALSE, "LED 11"=FALSE, "LED 12"=FALSE, "LED 13"=FALSE, "LED 14"=FALSE, "LED 15"=FALSE}  # LED Outputs
                  w197 = T24 {"PWM 0"=0, "PWM 1"=0, "PWM 2"=0, "PWM 3"=0, "PWM 4"=0, "PWM 5"=0, "PWM 6"=0, "PWM 7"=0, "PWM 8"=0, "PWM 9"=0, "PWM 10"=0}  # PWM Outputs
                  n89 = Tick Count (ms)() -> (millisecond timer value=w187:u32)
                  n90 = Wait (ms)(milliseconds to wait=u32 20) -> ()  [unwired: 1 out]
                  n91 = Quotient & Remainder(x=w187, y=u32 2000) -> (x-y*floor(x/y)=w185:u32)  [unwired: 1 out]
                  n92 = Greater?(x=w185, y=u32 1000) -> (0:w182:bool)
                  n93 = Cluster To Array(cluster=w197) -> (array=w207:u8[])
                  n94 = local read "Mode"() -> (w189:T6)
                  n95 = Cluster To Array(cluster=w210) -> (array=w227:bool[])
                  n96 = To Double Precision Float(number=w207) -> (double precision float=w206:dbl[])
                  n97 = Initialize Array(w182, 16 ("dimension size")) -> (w180:bool[])
                  n98 = Equal?(x=T6."Disconnected", y=w189) -> (x = y?=w183:bool)
                  n99 = feedback #1(w227) -> (w228:bool[])
                  n100 = feedback #2(w206) -> (w205:dbl[])
                  n101 = call-poly <vilib>:"NT Read Value.vi"("Default Value"=w228, "Name"="OICB - LEDs Out") -> ("Boolean Array"=w179:bool[])  [unwired: 8 in, 1 out]
                  n102 = feedback-in #1(w179) -> ()
                  n103 = call-poly <vilib>:"NT Read Value.vi"("Default Value"=w205, "Name"="OICD - PWMs Out") -> ("Numeric Array"=w196:dbl[])  [unwired: 8 in, 1 out]
                  n104 = feedback-in #2(w196) -> ()
                  n105 = To Unsigned Byte Integer(number=w196) -> (unsigned 8bit integer=w191:u8[])
                  n106 = Select(t=w180, s=w183, f=w179) -> (s? t:f=w178:bool[])
                  n107 = Index Array(array=w178) -> (element #1=w226:bool, element #2=w225:bool, element #3=w224:bool, element #4=w223:bool, element #5=w222:bool, element #6=w221:bool, element #7=w220:bool, element #8=w219:bool, element #9=w218:bool, element #10=w217:bool, element #11=w216:bool, element #12=w215:bool, element #13=w214:bool, element #14=w213:bool, element #15=w212:bool, element #16=w211:bool)  [unwired: 16 in]
                  n108 = Index Array(array=w191) -> (element #1=w204:u8, element #2=w203:u8, element #3=w202:u8, element #4=w201:u8, element #5=w200:u8, element #6=w199:u8, element #7=w198:u8, element #8=w195:u8, element #9=w194:u8, element #10=w193:u8, element #11=w192:u8)  [unwired: 11 in]
                  n109 = Bundle(cluster=w210, "LED 0"=w226, "LED 1"=w225, "LED 2"=w224, "LED 3"=w223, "LED 4"=w222, "LED 5"=w221, "LED 6"=w220, "LED 7"=w219, "LED 8"=w218, "LED 9"=w217, "LED 10"=w216, "LED 11"=w215, "LED 12"=w214, "LED 13"=w213, "LED 14"=w212, "LED 15"=w211) -> (w209:T23)
                  n110 = Bundle(cluster=w197, "PWM 0"=w204, "PWM 1"=w203, "PWM 2"=w202, "PWM 3"=w201, "PWM 4"=w200, "PWM 5"=w199, "PWM 6"=w198, "PWM 7"=w195, "PWM 8"=w194, "PWM 9"=w193, "PWM 10"=w192) -> (w190:T24)
                  n111 = call "Control Board - Update.vi"("error in (no error)"=w238, "PWM Outputs"=w190, "LED Outputs"=w209, "Control Board VISA Reference In"=w240) -> ("error out"=w237:errorcluster, "Analog Inputs"=w230:T25, "Switch Inputs"=w231:T26, "Control Board VISA Reference Out"=w239:refnum<visa-resource-name>)  [unwired: 4 in]
                  n112 = Cluster To Array(cluster=w231) -> (array=w234:bool[])
                  n113 = Cluster To Array(cluster=w230) -> (array=w235:u8[])
                  n114 = call-poly <vilib>:"NT Write Value.vi"("Boolean Array"=w234, "Name"="OICB - Switch In") -> ()  [unwired: 9 in, 1 out]
                  n115 = call-poly <vilib>:"NT Write Value.vi"("Numeric Array"=w235, "Name"="OICB - Analog In") -> ()  [unwired: 9 in, 1 out]
                }
                n116 = local write "Control Board Connection"(TRUE ("Connected")) -> ()
              }
              frame Error {
              }
            }
            n117 = call "Control Board - Close.vi"("error in (no error)"=w168, "VISA Refnum in"=w167) -> ()  [unwired: 9 in, 1 out]
          }
        }
        "Control Board Connection" <- FALSE
      }
    }
    frame Disabled {
    }
  }
  n118 = while {
    tunnel: w6 -> [w248]
    tunnel: w16 -> [w247]
    tunnel: w15 -> [w244]
    tunnel: w7 -> [w243]
    stop <- FALSE stop-if-true
    n119 = call <vilib>:"WPI_DashboardUpdateNames.vi"("Controls on Tab"=w247) -> ()  [unwired: 11 in]
    n120 = call <vilib>:"WPI_DashboardRetrieveStatusInfo.vi"("Vision"=w243, "Binding Refnum"=w248, "Window Mode Notifier"=w244, "TCP Cnx"="TCP") -> ("Power and Errors"=w249:T27, "Robot Metrics"=w252:T28, "Status Info"=w253:T29, "Control Info"=w250:T30, "Robot Mode"=w246:T6, "Process?"=w251:bool)  [unwired: 2 in]
    "Mode" <- w246
    n121 = case shown="True" w251 {
      tunnel: w253 -> [_ w312]
      tunnel: w252 -> [_ w311]
      tunnel: w250 -> [_ w310]
      tunnel: w249 -> [_ w309]
      tunnel: w246 -> [_ _]
      frame False {
        n122 = Wait (ms)(milliseconds to wait=u32 20) -> ()  [unwired: 1 out]
      }
      frame True {
        w275 = 12.0 ("y")
        # "swap motors to match\ncharts and include battery"
        n123 = Unbundle By Name(w310) -> ("Joystick Values"=w299:T31)  [unwired: 1 out]
        n124 = Unbundle By Name(w309) -> ()  [unwired: 2 out]
        n125 = Unbundle By Name(w311) -> ()  [unwired: 1 out]
        n126 = Unbundle By Name(w312) -> ("Battery V"=w300:dbl)  [unwired: 1 out]
        n127 = call-poly <vilib>:"NT Read Value.vi"("Name"="Left Drive Speed") -> ("Numeric"=→"Left Drive Speed":dbl)  [unwired: 9 in, 1 out]
        n128 = call-poly <vilib>:"NT Read Value.vi"("Name"="Right Drive Speed") -> ("Numeric"=→"Right Drive Speed":dbl)  [unwired: 9 in, 1 out]
        n129 = call-poly <vilib>:"NT Read Value.vi"("Name"="Robot Direction") -> ("Numeric"=→"Robot Direction":dbl)  [unwired: 9 in, 1 out]
        n130 = call-poly <vilib>:"NT Read Value.vi"("Name"="RobotDrive Motors") -> ("Numeric Array"=w289:dbl[])  [unwired: 9 in, 1 out]
        n131 = Index Array(array=w289, index #1=1, index #4=0) -> (element #1=w304:dbl, element #2=w305:dbl, element #3=w303:dbl, element #4=w308:dbl)  [unwired: 2 in]
        n132 = Index Array(array=w299) -> (element #1=w298:T32, element #2=w294:T32)  [unwired: 2 in]
        n133 = call "Prepare Joystick Data for Displays.vi"("Joystick Values"=w294) -> ("Buttons"=→"JS2 Buttons":T33, "Z Axis"=→"JS2 Z":dbl, "Cartesian Data"=→"JS2 Graph":cluster{"X axis":dbl, "X axis":dbl}[])  [unwired: 8 in]
        n134 = call "Prepare Joystick Data for Displays.vi"("Joystick Values"=w298) -> ("Buttons"=→"JS1 Buttons":T33, "Z Axis"=→"JS1 Z":dbl, "Cartesian Data"=→"JS1 Graph":cluster{"X axis":dbl, "X axis":dbl}[])  [unwired: 8 in]
        n135 = Bundle("Numeric"=w303, "Numeric"=w304) -> (→"MotorChart R" →"MotorSliders R":cluster{"Numeric":dbl, "Numeric":dbl})  [unwired: 1 in]
        n136 = Bundle("Numeric"=w305, "Numeric"=w308, "Battery V"=w300) -> (→"MotorChart L" →"MotorSliders L":T3)  [unwired: 1 in]
        n137 = call-poly <vilib>:"NT Read Value.vi"("Name"="Arm - Mode") -> ("String"=→"Arm Mode":string)  [unwired: 9 in, 1 out]
        n138 = call-poly <vilib>:"NT Read Value.vi"("Name"="Arm Unlocked?") -> ("Boolean"=→"Arm Lock State":bool)  [unwired: 9 in, 1 out]
        n139 = call-poly <vilib>:"NT Read Value.vi"("Name"="Air Pressure") -> ("Numeric"=→"Air Presure":dbl)  [unwired: 9 in, 1 out]
        n140 = call-poly <vilib>:"NT Read Value.vi"("Name"="Arm - Set Angle") -> ("Numeric"=w280:dbl)  [unwired: 9 in, 1 out]
        n141 = call-poly <vilib>:"NT Read Value.vi"("Name"="Arm - Current Angle") -> ("Numeric"=w279:dbl)  [unwired: 9 in, 1 out]
        n142 = call-poly <vilib>:"NT Read Value.vi"("Default Value"=-1.0, "Name"="Front Distance") -> ("Numeric"=w268:dbl)  [unwired: 8 in, 1 out]
        n143 = call-poly <vilib>:"NT Read Value.vi"("Name"="Autonomous Mode") -> ("Numeric"=w270:dbl)  [unwired: 9 in, 1 out]
        n144 = Greater Or Equal To 0?(x=w268) -> (x >= 0?=w265:bool)
        n145 = Bundle(cluster=cluster{dbl, dbl} {90.0, 90.0} ("Arm Angles"), w280, w279) -> (→"Arm Information":cluster{dbl, dbl})
        n146 = Divide(x=w268, y=w275) -> (x/y=→"Front Distance":dbl)
        n147 = To Unsigned Byte Integer(number=w270) -> (unsigned 8bit integer=→"Autonomous Selection":u8)
        n148 = Quotient & Remainder(x=w268, y=w275) -> (x-y*floor(x/y)=w274:dbl, floor(x/y)=w273:dbl)
        n149 = Format Into String(format string="%d ft. %d in" ("initial string"), w273, w274) -> (resulting string=w267:string)  [unwired: 2 in, 1 out]
        n150 = Select(t=w267, s=w265, f="No Value") -> (s? t:f=→"Distance":string)
      }
    }
  }
  n151 = while {
    tunnel: w31 -> [w323]
    shift-right: [w322] -> _
    shift-left: w30 -> [w321]
    tunnel: [w320] -> _
    tunnel: w29 -> [w319]
    tunnel: w28 -> [w318]
    tunnel: w27 -> [_]
    tunnel: w24 -> [w317]
    tunnel: w9 -> [w316]
    tunnel: w8 -> [w315]
    shift-right: [w314] -> _
    shift-left: _ -> [w313]
    i -> [w320]
    stop <- FALSE stop-if-true
    n152 = event shown="[0] Timeout" {
      selector: w318 -> [_ _ _ _ _ _ _ _ _ _ _ _ _ _ _ _ _ _]
      dyn-events: _ -> [_ _ _ _ _ _ _ _ _ _ _ _ _ _ _ _ _ _]
      timeout: u32 60 ("milliseconds to wait") -> [_ _ _ _ _ _ _ _ _ _ _ _ _ _ _ _ _ _]
      tunnel: w319 -> [w336 _ _ _ _ _ _ _ _ _ _ _ _ _ _ _ _ _]
      tunnel: "Test Tree" -> [_ _ _ _ _ _ _ _ _ w548 w557 w560 w565 w574 _ _ _ _]
      tunnel: w323 -> [_ w374 _ _ _ _ _ _ _ _ _ _ _ _ _ _ _ _]
      tunnel: [w333 w373 w477 w483 w495 w507 w515 w521 w534 w547 w555 w559 w564 w573 w580 w582 w589 w597] -> w322
      tunnel: w321 -> [w333 w373 w477 w483 w495 w507 w515 w521 w534 w547 w555 w559 w564 w573 w580 w582 w589 w597]
      tunnel: w317 -> [_ _ _ _ _ _ _ _ _ _ _ _ _ _ _ _ _ _]
      tunnel: w316 -> [_ _ _ _ _ _ _ _ _ _ _ _ _ _ _ _ _ _]
      tunnel: w315 -> [w328 _ _ _ w493 _ _ _ _ _ _ _ _ _ _ _ _ _]
      tunnel: [w327 w372 w476 w482 w491 w501 w512 w520 w533 w546 w554 w558 w563 w572 w578 w581 w585 w598] -> w314
      tunnel: w313 -> [w327 w372 w476 w482 w491 _ _ w520 w533 w546 w554 w558 w563 w572 w578 w581 w585 w598]
      event Timeout {
        n153 = event-data() -> ()  [unwired: 1 in, 1 out]
        n154 = local read "Mode"() -> (w330:T6)
        n155 = call <vilib>:"NT Read String.vi"("Name"="/TestMode/TestName") -> ("String"=w339:string)  [unwired: 9 in, 1 out]
        n156 = case shown="\"Test\"" "Dashboard Tab" {
          tunnel: w336 -> [_ w350 _ _]
          tunnel: "/TestMode/Automatic/" ("Name Pattern") -> [_ w349 _ _]
          tunnel: T34 [{"Operation"=enum."Clear", "Color Box"=14013909}, {"Operation"=enum."Clear", "Color Box"=14013909}, {"Operation"=enum."Clear", "Color Box"=14013909}, {"Operation"=enum."Clear", "Color Box"=14013909}, {"Operation"=enum."Update", "Color Box"=14013909}, {"Operation"=enum."Update", "Color Box"=16777215}, {"Operation"=enum."Clear", "Color Box"=14013909}, {"Operation"=enum."Clear", "Color Box"=14013909}, {"Operation"=enum."Clear", "Color Box"=14013909}] -> [_ w342 _ w359]
          tunnel: w330 -> [_ w341 _ w358]
          tunnel: u32[] [15790320, 15790320, 15790320, 15790320, 16777215, 16777215, 15790320, 15790320, 15790320] -> [_ _ _ w364]
          tunnel: w328 -> [_ _ _ w352]
          frame "Garnet Squadron", Default {
          }
          frame "Test" {
            w348 = -2 ("Active Item:Row Number")
            n157 = Index Array(array=w342, index=w341) -> (element=w343:T36)
            n158 = Unbundle(w343) -> ("Operation"=w344:enum16{"Update", "Clear"}, "Color Box"=w345:u32)
            n159 = call <vilib>:"NT Read and Format Entries as Tree.vi"("Operation"=w344, "Name Pattern"=w349, "Tree Refnum"=w350) -> ()  [unwired: 7 in, 2 out]
            n160 = property on="Test Tree" class="Tree (strict)"("Active Item Row Number"=w348, "ActiveColNum"=w348, "CellBG"=w345, "Active Item Row Number"=-1 ("Active Item:Row Number"), "CellBG"=u32 5789784 ("Color Box")) -> ()  [unwired: 2 in, 2 out]
          }
          frame "Variables" {
            n161 = control-ref of="Tree"() -> (w351:refnum<vi>)
            n162 = call <vilib>:"NT Read and Format Entries as Tree.vi"("Tree Refnum"=w351) -> ()  [unwired: 9 in, 2 out]
          }
          frame "Commands" {
            w360 = u32 5789784 ("Color Box")
            w361 = T37 {"Row"=-1, "Column"=-2} ("Active Cell:Active Cell")
            w363 = T37 {"Row"=-2, "Column"=-2} ("Active Cell:Active Cell")
            n163 = Index Array(array=w364, index=w358) -> (element=w362:u32)
            n164 = Index Array(array=w359, index=w358) -> (element=w357:T36)
            n165 = Unbundle(w357) -> ("Operation"=w356:enum16{"Update", "Clear"})  [unwired: 1 out]
            n166 = local read "Command Selection"() -> (w355:i32)
            n167 = property on="Command Selection" class="MCListbox (strict)"("ActiveCell"=w363, "CellBG"=w362, "ActiveCell"=w361, "CellBG"=w360) -> ()  [unwired: 2 in, 2 out]
            n168 = call <vilib>:"WPI_DashboardUpdate RPC Info.vi"("Operation"=w356) -> ("update"=w354:bool, "commands"=w353:string[][])  [unwired: 9 in]
            n169 = property on="Command Selection" class="MCListbox (strict)"("ItemNames"=w353) -> ()  [unwired: 2 in, 2 out]
            n170 = property on="Command Params" class="Tbl (strict)"("Active Cell"=w363, "Cell BG Color"=w362, "Active Cell"=w361, "Cell BG Color"=w360) -> ()  [unwired: 2 in, 2 out]
            n171 = call <vilib>:"WPI_DashboardUpdate Command Params.vi"("Update"=w354, "NewVal"=w355, "Commands"=w353, "Param Tbl"=w352) -> ()  [unwired: 7 in, 1 out]
          }
        }
        n172 = case shown="\"\"" w339 {
          tunnel: "/TestMode/TestProgress" ("Name") -> [w366 _]
          tunnel: "/TestMode/TestProgressText" ("Name") -> [w365 _]
          frame Default {
            n173 = call <vilib>:"NT Read Number.vi"("Name"=w366) -> ("Numeric"=w367:dbl)  [unwired: 9 in, 1 out]
            n174 = call <vilib>:"NT Read String.vi"("Name"=w365) -> ("String"=w368:string)  [unwired: 9 in, 1 out]
            n175 = Bundle("Numeric"=w367, "String"=w368) -> (→"Progress":cluster{"Numeric":dbl, "String":string})  [unwired: 1 in]
          }
          frame "" {
            n176 = property on="Progress" class="Clust (strict)"("Visible"=FALSE) -> ()  [unwired: 2 in, 2 out]
            n177 = local write "Test Name"(u16 0) -> ()
          }
        }
        n178 = call <vilib>:"Connextion Info.vi"() -> ("Connected"=→"Network Table Connection":bool)  [unwired: 10 in, 1 out]
      }
      event "Test Tree": Value Change {
        # "Show appropriate\ncontrols"
        n179 = event-data() -> ("CtlRef"=w377:refnum<vi>, "NewVal"=w375:string)  [unwired: 1 in]
        n180 = call <vilib>:"WPI_UtilitiesGetTreeIOName.vi"("NewVal"=w375, "TreeControl in"=w377) -> ("I/O Name"=w378:string)  [unwired: 9 in]
        n181 = case shown="\"Analog Out\", \"Motor\", \"PWM\"" w378 {
          selector: w378 -> [_ w385 _ w407 w416 _]
          tunnel: w375 -> [_ _ w404 w406 _ w423]
          tunnel: w374 -> [_ _ _ _ _ w422]
          frame Default {
            w380 = FALSE ("Visible")
            w379 = FALSE ("Visible")
            n182 = property on="Motor" class="Clust (strict)"("Visible"=w379) -> ()  [unwired: 2 in, 2 out]
            n183 = property on="Test Ring" class="Ring (strict)"("Visible"=w379) -> ()  [unwired: 2 in, 2 out]
            n184 = property on="Rev/Fwd" class="Clust (strict)"("Visible"=w380) -> ()  [unwired: 2 in, 2 out]
            n185 = property on="On/Off" class="Bool (strict)"("Visible"=w380) -> ()  [unwired: 2 in, 2 out]
            n186 = property on="Test Slider" class="Slide (strict)"("Visible"=w380) -> ()  [unwired: 2 in, 2 out]
          }
          frame "Analog Out", "Motor", "PWM" {
            w386 = FALSE ("Visible")
            n187 = case shown="\"Analog Out\"" w385 {
              tunnel: [1.0 ("Value") -1.0 ("Value") 0.0 ("Value")] -> w384
              tunnel: [255.0 ("Value") 1.0 ("Value") 5.0 ("Value")] -> w383
              tunnel: [128.0 ("Value") 0.0 ("Value") 0.0 ("Value")] -> w382
              tunnel: [64.0 ("Value") 0.5 ("Value") 1.0 ("Value")] -> w381
              frame "PWM" {
              }
              frame "Motor", Default {
              }
              frame "Analog Out" {
              }
            }
            n188 = property on="Motor" class="Clust (strict)"("Visible"=TRUE) -> ()  [unwired: 2 in, 2 out]
            n189 = property on="Value" class="Slide (strict)"("Value"=w382, "Scale.Minimum"=w384, "Scale.Maximum"=w383, "Scale.Increment"=w381) -> ()  [unwired: 2 in, 2 out]
            n190 = property on="On/Off" class="Bool (strict)"("Visible"=w386) -> ()  [unwired: 2 in, 2 out]
            n191 = property on="Test Slider" class="Slide (strict)"("Visible"=w386) -> ()  [unwired: 2 in, 2 out]
            n192 = property on="Test Ring" class="Ring (strict)"("Visible"=w386) -> ()  [unwired: 2 in, 2 out]
            n193 = property on="Rev/Fwd" class="Clust (strict)"("Visible"=w386) -> ()  [unwired: 2 in, 2 out]
          }
          frame "Servo" {
            w402 = FALSE ("Visible")
            n194 = call <vilib>:"NT Read Number.vi"("Name"=w404) -> ("Numeric"=w403:dbl)  [unwired: 9 in, 1 out]
            n195 = property on="Test Slider" class="Slide (strict)"("Visible"=TRUE, "Scale.Maximum"=170.0 ("Scale.Range:Maximum")) -> ()  [unwired: 2 in, 2 out]
            n196 = local write "Test Slider"(w403) -> ()
            n197 = property on="Motor" class="Clust (strict)"("Visible"=w402) -> ()  [unwired: 2 in, 2 out]
            n198 = property on="Rev/Fwd" class="Clust (strict)"("Visible"=w402) -> ()  [unwired: 2 in, 2 out]
            n199 = property on="On/Off" class="Bool (strict)"("Visible"=w402) -> ()  [unwired: 2 in, 2 out]
            n200 = property on="Test Ring" class="Ring (strict)"("Visible"=w402) -> ()  [unwired: 2 in, 2 out]
          }
          frame "Relay", "Solenoid" {
            w405 = FALSE ("Visible")
            n201 = property on="Motor" class="Clust (strict)"("Visible"=w405) -> ()  [unwired: 2 in, 2 out]
            n202 = property on="Test Slider" class="Slide (strict)"("Visible"=w405) -> ()  [unwired: 2 in, 2 out]
            n203 = Search and Replace String(input string=w406, search string="/Value  **", replace string="/Direction") -> (result string=w412:string)  [unwired: 5 in, 3 out]
            n204 = property on="Test Ring" class="Ring (strict)"("Visible"=w405) -> ()  [unwired: 2 in, 2 out]
            n205 = call <vilib>:"NT Read String.vi"("Name"=w412) -> ("String"=w410:string)  [unwired: 9 in, 1 out]
            n206 = Equal?(x="Both directions", y=w410) -> (x = y?=w408:bool)
            n207 = Not(x=w408) -> (.not. x?=w409:bool)
            n208 = property on="Rev/Fwd" class="Clust (strict)"("Visible"=w408) -> ()  [unwired: 2 in, 2 out]
            n209 = property on="On/Off" class="Bool (strict)"("Visible"=w409, "Caption.Text"=w407) -> ()  [unwired: 2 in, 2 out]
          }
          frame "Compressor", "Digital Out" {
            w415 = FALSE ("Visible")
            # "Get direction and finish"
            n210 = property on="Motor" class="Clust (strict)"("Visible"=w415) -> ()  [unwired: 2 in, 2 out]
            n211 = property on="Test Slider" class="Slide (strict)"("Visible"=w415) -> ()  [unwired: 2 in, 2 out]
            n212 = property on="Test Ring" class="Ring (strict)"("Visible"=w415) -> ()  [unwired: 2 in, 2 out]
            n213 = property on="On/Off" class="Bool (strict)"("Visible"=TRUE, "Caption.Text"=w416) -> ()  [unwired: 2 in, 2 out]
            n214 = property on="Rev/Fwd" class="Clust (strict)"("Visible"=FALSE) -> ()  [unwired: 2 in, 2 out]
          }
          frame "Camera" {
            n215 = call <vilib>:"Get Last Path Segment.vi"("String in"=w423) -> ("String out"=w424:string)  [unwired: 10 in]
            n216 = property on="On/Off" class="Bool (strict)"("Visible"=FALSE) -> ()  [unwired: 2 in, 2 out]
            n217 = property on="Motor" class="Clust (strict)"("Visible"=FALSE) -> ()  [unwired: 2 in, 2 out]
            n218 = property on="Rev/Fwd" class="Clust (strict)"("Visible"=FALSE) -> ()  [unwired: 2 in, 2 out]
            n219 = case shown="\"White Balance  **\"" w424 {
              tunnel: w423 -> [w430 w439 w448 w457 w466 _ w472]
              tunnel: w422 -> [w428 w436 w445 w454 w463 _ _]
              frame "Size  **" {
                n220 = Index Array(array=w428) -> (element=w427:cluster{string[]})  [unwired: 1 in]
                n221 = call <vilib>:"NT Read String.vi"("Name"=w430) -> ("String"=w429:string)  [unwired: 9 in, 1 out]
                n222 = Unbundle(w427) -> (w425:string[])
                n223 = Match First String(2:w425, 3:w429) -> (0:w426:i32)  [unwired: 1 out]
                n224 = property on="Test Ring" class="Ring (strict)"("Value"=w426, "Strings []"=w425) -> ()  [unwired: 2 in, 2 out]
                n225 = property on="Test Ring" class="Ring (strict)"("Visible"=TRUE) -> ()  [unwired: 2 in, 2 out]
                n226 = property on="Test Slider" class="Slide (strict)"("Visible"=FALSE) -> ()  [unwired: 2 in, 2 out]
              }
              frame "White Balance  **" {
                n227 = Index Array(array=w436, index=1) -> (element=w437:cluster{string[]})
                n228 = call <vilib>:"NT Read String.vi"("Name"=w439) -> ("String"=w438:string)  [unwired: 9 in, 1 out]
                n229 = Unbundle(w437) -> (w434:string[])
                n230 = Match First String(2:w434, 3:w438) -> (0:w433:i32)  [unwired: 1 out]
                n231 = property on="Test Ring" class="Ring (strict)"("Value"=w433, "Strings []"=w434) -> ()  [unwired: 2 in, 2 out]
                n232 = property on="Test Ring" class="Ring (strict)"("Visible"=TRUE) -> ()  [unwired: 2 in, 2 out]
                n233 = property on="Test Slider" class="Slide (strict)"("Visible"=FALSE) -> ()  [unwired: 2 in, 2 out]
              }
              frame "Exposure  **" {
                n234 = Index Array(array=w445, index=2) -> (element=w446:cluster{string[]})
                n235 = call <vilib>:"NT Read String.vi"("Name"=w448) -> ("String"=w447:string)  [unwired: 9 in, 1 out]
                n236 = Unbundle(w446) -> (w442:string[])
                n237 = Match First String(2:w442, 3:w447) -> (0:w443:i32)  [unwired: 1 out]
                n238 = property on="Test Ring" class="Ring (strict)"("Value"=w443, "Strings []"=w442) -> ()  [unwired: 2 in, 2 out]
                n239 = property on="Test Ring" class="Ring (strict)"("Visible"=TRUE) -> ()  [unwired: 2 in, 2 out]
                n240 = property on="Test Slider" class="Slide (strict)"("Visible"=FALSE) -> ()  [unwired: 2 in, 2 out]
              }
              frame "Exposure Priority  **" {
                n241 = Index Array(array=w454, index=3) -> (element=w455:cluster{string[]})
                n242 = call <vilib>:"NT Read String.vi"("Name"=w457) -> ("String"=w456:string)  [unwired: 9 in, 1 out]
                n243 = Unbundle(w455) -> (w451:string[])
                n244 = Match First String(2:w451, 3:w456) -> (0:w452:i32)  [unwired: 1 out]
                n245 = property on="Test Ring" class="Ring (strict)"("Value"=w452, "Strings []"=w451) -> ()  [unwired: 2 in, 2 out]
                n246 = property on="Test Ring" class="Ring (strict)"("Visible"=TRUE) -> ()  [unwired: 2 in, 2 out]
                n247 = property on="Test Slider" class="Slide (strict)"("Visible"=FALSE) -> ()  [unwired: 2 in, 2 out]
              }
              frame "Color Enable  **" {
                n248 = Index Array(array=w463, index=4) -> (element=w464:cluster{string[]})
                n249 = call <vilib>:"NT Read String.vi"("Name"=w466) -> ("String"=w465:string)  [unwired: 9 in, 1 out]
                n250 = Unbundle(w464) -> (w460:string[])
                n251 = Match First String(2:w460, 3:w465) -> (0:w461:i32)  [unwired: 1 out]
                n252 = property on="Test Ring" class="Ring (strict)"("Value"=w461, "Strings []"=w460) -> ()  [unwired: 2 in, 2 out]
                n253 = property on="Test Ring" class="Ring (strict)"("Visible"=TRUE) -> ()  [unwired: 2 in, 2 out]
                n254 = property on="Test Slider" class="Slide (strict)"("Visible"=FALSE) -> ()  [unwired: 2 in, 2 out]
              }
              frame Default {
                n255 = property on="Test Ring" class="Ring (strict)"("Visible"=FALSE) -> ()  [unwired: 2 in, 2 out]
                n256 = property on="Test Slider" class="Slide (strict)"("Visible"=FALSE) -> ()  [unwired: 2 in, 2 out]
              }
              frame "Brightness  **", "Color Level  **", "Compression  **", "FPS  **", "Sharpness  **" {
                n257 = call <vilib>:"NT Read Number.vi"("Name"=w472) -> ("Numeric"=w471:dbl)  [unwired: 9 in, 1 out]
                n258 = local write "Test Slider"(w471) -> ()
                n259 = property on="Test Slider" class="Slide (strict)"("Visible"=TRUE, "Scale.Maximum"=100.0 ("Scale.Range:Maximum")) -> ()  [unwired: 2 in, 2 out]
                n260 = property on="Test Ring" class="Ring (strict)"("Visible"=FALSE) -> ()  [unwired: 2 in, 2 out]
              }
            }
          }
        }
        n261 = property on="Progress" class="Clust (strict)"("Visible"=FALSE) -> ()  [unwired: 2 in, 2 out]
      }
      event "Test Name": Mouse Enter {
        # "Populate the ring with the list of tests"
        n262 = event-data() -> ()  [unwired: 1 in, 1 out]
        n263 = call <vilib>:"NT Read String Array.vi"("Name"="/TestMode/TestList") -> ("String Array"=w481:string[])  [unwired: 9 in, 1 out]
        n264 = Build Array (concatenate)("Select the test to run...", w481) -> (w480:string[])
        n265 = property on="Test Name" class="Ring (strict)"("Strings []"=w480) -> ()  [unwired: 2 in, 2 out]
      }
      event "Test Name": Value Change {
        w484 = FALSE ("Visible")
        # "Tell the robot the test name to run"
        n266 = event-data() -> ("NewVal"=w488:u16)  [unwired: 1 in]
        n267 = property on="Test Name" class="Ring (strict)"() -> ("Strings []"=w489:string[])  [unwired: 2 in, 2 out]
        n268 = local write "Progress"(T7 {"Test Progress"=0, "Test Progress Text"=""} ("Progress")) -> ()
        n269 = Index Array(array=w489, index=w488) -> (element=w487:string)
        n270 = call <vilib>:"NT Write String.vi"("String"=w487, "Name"="/TestMode/TestName") -> ()  [unwired: 9 in, 1 out]
        n271 = property on="Progress" class="Clust (strict)"("Visible"=TRUE) -> ()  [unwired: 2 in, 2 out]
        n272 = property on="Motor" class="Clust (strict)"("Visible"=w484) -> ()  [unwired: 2 in, 2 out]
        n273 = property on="Test Slider" class="Slide (strict)"("Visible"=w484) -> ()  [unwired: 2 in, 2 out]
        n274 = property on="On/Off" class="Bool (strict)"("Visible"=w484) -> ()  [unwired: 2 in, 2 out]
        n275 = property on="Rev/Fwd" class="Clust (strict)"("Visible"=w484) -> ()  [unwired: 2 in, 2 out]
        n276 = property on="Test Ring" class="Ring (strict)"("Visible"=w484) -> ()  [unwired: 2 in, 2 out]
      }
      event "Command Selection": Value Change {
        # "Get the params and show in table"
        n277 = event-data() -> ("NewVal"=w494:i32)  [unwired: 1 in]
        n278 = property on="Command Selection" class="MCListbox (strict)"() -> ("ItemNames"=w492:string[][])  [unwired: 2 in, 2 out]
        n279 = call <vilib>:"WPI_DashboardUpdate Command Params.vi"("NewVal"=w494, "Commands"=w492, "Param Tbl"=w493) -> ()  [unwired: 8 in, 1 out]
      }
      event "Execute Command": Value Change {
        # "Started one, Unique ID holds\nresponse"
        n280 = event-data() -> ()  [unwired: 1 in, 1 out]
        n281 = property on="Command Selection" class="MCListbox (strict)"() -> ("ItemNames"=w506:string[][])  [unwired: 2 in, 2 out]
        n282 = Index Array(array=w506, index (row)="Command Selection", index (col)=0) -> (element=w504:string)
        n283 = call <vilib>:"Invoke Commands.vi"("Command Params"="Command Params", "Function Name"=w504) -> ("Params"=w500:u8, "Started"=w499:bool)  [unwired: 7 in, 1 out]
        n284 = Array Subset(array="Command Params", length (row)=w500) -> (w501:string[][])  [unwired: 3 in]
        n285 = Select(t="Executing" ("Cmd Status"), s=w499, f="" ("Cmd Status")) -> (s? t:f=→"Cmd Status":string)
      }
      event "Command Selection": Double Click {
        n286 = event-data() -> ("Row"=w516:i32)  [unwired: 1 in]
        n287 = property on="Command Selection" class="MCListbox (strict)"() -> ("ItemNames"=w519:string[][])  [unwired: 2 in, 2 out]
        n288 = local read "Command Params"() -> (w514:string[][])
        n289 = Index Array(array=w519, index (row)=w516, index (col)=0) -> (element=w517:string)
        n290 = call <vilib>:"Invoke Commands.vi"("Command Params"=w514, "Function Name"=w517) -> ("Params"=w513:u8, "Started"=w508:bool)  [unwired: 7 in, 1 out]
        n291 = Array Subset(array=w514, length (row)=w513) -> (w512:string[][])  [unwired: 3 in]
        n292 = Select(t="Executing" ("Cmd Status"), s=w508, f="" ("Cmd Status")) -> (s? t:f=w509:string)
        n293 = local write "Cmd Status"(w509) -> ()
      }
      event "CheckList": Double Click {
        # "Shift clears all"
        # "Update symbols on the listbox"
        n294 = event-data() -> ("PlatMods.Shift"=w522:bool, "Row"=w524:i32)  [unwired: 1 in]
        n295 = case shown="True" w522 {
          tunnel: w524 -> [w528 _]
          tunnel: 1 -> [w527 _]
          frame False {
            n296 = property on="CheckList" class="LstBox (strict)"() -> ("Item Symbols"=w526:i32[])  [unwired: 2 in, 2 out]
            n297 = Replace Array Subset(array=w526, new element=w527, index=w528) -> (w525:i32[])
            n298 = property on="CheckList" class="LstBox (strict)"("Item Symbols"=w525) -> ()  [unwired: 2 in, 2 out]
          }
          frame True {
            w529 = 0 ("Top Row")
            n299 = property on="CheckList" class="LstBox (strict)"() -> ("Number of Rows"=w531:u32)  [unwired: 2 in, 2 out]
            n300 = Initialize Array(0, w531) -> (w530:i32[])
            n301 = property on="CheckList" class="LstBox (strict)"("Top Row"=w529, "Value"=w529, "Item Symbols"=w530) -> ()  [unwired: 2 in, 2 out]
          }
        }
      }
      event "CheckList": Key Down {
        # "Update symbols on the listbox\nLeft and right keys check and uncheck"
        n302 = event-data() -> ("VKey"=w536:T35)  [unwired: 1 in]
        n303 = case shown="\"Left\", \"Right\"" w536 {
          selector: w536 -> [w541 _]
          tunnel: eventvkey."Left" ("VKey") -> [w539 _]
          frame "Left", "Right" {
            n304 = Equal?(x=w539, y=w541) -> (x = y?=w540:bool)
            n305 = Select(t=0, s=w540, f=1) -> (s? t:f=w542:i32)
            n306 = property on="CheckList" class="LstBox (strict)"() -> ("Item Symbols"=w545:i32[])  [unwired: 2 in, 2 out]
            n307 = Replace Array Subset(array=w545, new element=w542, index="CheckList") -> (w544:i32[])
            n308 = property on="CheckList" class="LstBox (strict)"("Item Symbols"=w544) -> ()  [unwired: 2 in, 2 out]
          }
          frame Default {
          }
        }
      }
      event "Motor.Enable": Value Change {
        # "When the test mode otor enable helper is set, update that\ntree row item's value"
        n309 = event-data() -> ("NewVal"=w552:bool)  [unwired: 1 in]
        n310 = Unbundle("Motor") -> ("Value"=w551:dbl)  [unwired: 1 out]
        n311 = Select(t=w551, s=w552, f=0.0) -> (s? t:f=w549:dbl)
        n312 = call <vilib>:"NT Write Number.vi"("Numeric"=w549, "Name"=w548) -> ()  [unwired: 9 in, 1 out]
      }
      event "Test Slider": Value Change {
        # "When the test mode slider helper is set, update that\ntree row item's value"
        n313 = event-data() -> ("NewVal"=w556:dbl)  [unwired: 1 in]
        n314 = call <vilib>:"NT Write Number.vi"("Numeric"=w556, "Name"=w557) -> ()  [unwired: 9 in, 1 out]
      }
      event "On/Off": Value Change {
        # "When the test mode on/off helper value is set, update that\ntree row item's value"
        n315 = event-data() -> ("NewVal"=w562:bool)  [unwired: 1 in]
        n316 = Boolean To (0,1)(Boolean=w562) -> (0, 1=w561:i16)
        n317 = call <vilib>:"NT Write Number.vi"("Numeric"=w561, "Name"=w560) -> ()  [unwired: 9 in, 1 out]
      }
      event "Rev/Fwd": Value Change {
        # "When the test mode helper value for relays is set, update that\ntree row item's value"
        n318 = event-data() -> ("NewVal.Forward"=w571:bool, "NewVal.Reverse"=w570:bool)  [unwired: 1 in]
        n319 = Boolean To (0,1)(Boolean=w571) -> (0, 1=w567:i16)
        n320 = Boolean To (0,1)(Boolean=w570) -> (0, 1=w569:i16)
        n321 = Negate(x=w569) -> (-x=w568:i16)
        n322 = Add(x=w567, y=w568) -> (x+y=w566:i16)
        n323 = call <vilib>:"NT Write Number.vi"("Numeric"=w566, "Name"=w565) -> ()  [unwired: 9 in, 1 out]
      }
      event "Test Ring": Value Change {
        # "When a test mode helper value is selected from the ring,\nset the tree item's variable to the string value"
        n324 = event-data() -> ("NewVal"=w576:u16)  [unwired: 1 in]
        n325 = property on="Test Ring" class="Ring (strict)"() -> ("Strings []"=w577:string[])  [unwired: 2 in, 2 out]
        n326 = Index Array(array=w577, index=w576) -> (element=w575:string)
        n327 = call <vilib>:"NT Write String.vi"("String"=w575, "Name"=w574) -> ()  [unwired: 9 in, 1 out]
      }
      event Panel Close {
        # "Playback window has been closed, abort"
        n328 = event-data() -> ()  [unwired: 1 in, 4 out]
        n329 = global write "WPI_DashboardLogging Global.vi" "Recording"(enum32{"Stop", "Record", "Playback"}."Stop" ("Rec Mode")) -> ()
      }
      event Panel Close {
        # "Abort playback window and ourself"
        n330 = event-data() -> ()  [unwired: 1 in, 4 out]
        n331 = invoke class="VI" method="FP.Close"() -> (reference out=w584:refnum<vi>)  [unwired: 3 in, 2 out]
        n332 = invoke class="VI" method="Abort VI"(reference=w584) -> (error out=w583:errorcluster)  [unwired: 2 in, 2 out]
        n333 = invoke class="VI" method="Abort VI"(error in=w583) -> ()  [unwired: 2 in, 3 out]
      }
      event User Event {
        n334 = event-data() -> ("IDs"=w592:cluster{"RPC field ID":u16, "Unique ID":u16}, "String"=w591:string)  [unwired: 1 in]
        n335 = Bundle("IDs"=w592, "String"=w591) -> (w590:T13)  [unwired: 1 in]
        n336 = call <vilib>:"Retrieve RPC Response.vi"("RPC Response"=w590) -> ("Output"=w587:string[][])  [unwired: 10 in]
        n337 = Build Array (concatenate)(w585, w587) -> (w586:string[][])
        n338 = local write "Command Params"(w586) -> ()
        n339 = local write "Cmd Status"("" ("Cmd Status")) -> ()
      }
      event "Tree": Double Click {
        n340 = event-data() -> ("PlatMods"=w596:T38, "Tag"=w595:string)  [unwired: 1 in]
        n341 = Unbundle(w596) -> ("Shift"=w594:bool)  [unwired: 4 out]
        n342 = Not(x=w594) -> (.not. x?=w593:bool)
        n343 = call <vilib>:"NT Update Persistence.vi"("Persistence"=w593, "Name"=w595) -> ()  [unwired: 9 in, 1 out]
      }
    }
  }
  n344 = local write "Dashboard Tab"(T1."Garnet Squadron" ("Dashboard Tab")) -> ()
  n345 = property on="On/Off" class="Bool (strict)"("Visible"=w17) -> ()  [unwired: 2 in, 2 out]
  n346 = property on="Motor" class="Clust (strict)"("Visible"=w17) -> ()  [unwired: 2 in, 2 out]
  n347 = property on="Progress" class="Clust (strict)"("Visible"=w17) -> ()  [unwired: 2 in, 2 out]
  n348 = property on="Test Ring" class="Ring (strict)"("Visible"=w17) -> ()  [unwired: 2 in, 2 out]
  n349 = property on="Rev/Fwd" class="Clust (strict)"("Visible"=w17) -> ()  [unwired: 2 in, 2 out]
  n350 = local write "DB Camera Config"(w17) -> ()
  n351 = while {
    tunnel: u16 1741 ("timeout ms (25000)") -> [w600]
    stop <- FALSE stop-if-true
    n352 = TCP Create Listener(10:w600) -> (0:w599:errorcluster, 3:w601:refnum<k5>)  [unwired: 4 in, 1 out]
    n353 = case shown="No Error" w599 {
      selector: w599 -> [w603 _]
      tunnel: w601 -> [w604 _]
      frame No Error {
        n354 = while {
          tunnel: w604 -> [w607]
          tunnel: w603 -> [w606]
          stop <- FALSE stop-if-true
          n355 = TCP Wait On Listener(8:w606, 11:w607) -> (0:w608:errorcluster, 4:w609:refnum<k5>)  [unwired: 2 in, 3 out]
          n356 = local write "TCP"(w609) -> ()
          n357 = case shown="No Error" w608 {
            frame No Error {
            }
            frame Error {
              n358 = Wait (ms)(milliseconds to wait=u32 1000) -> ()  [unwired: 1 out]
            }
          }
        }
      }
      frame Error {
        n359 = Wait (ms)(milliseconds to wait=u32 1000) -> ()  [unwired: 1 out]
      }
    }
  }
  n360 = local write "Command Params"(string[][] [] ("Command Params")) -> ()
  n361 = local write "Command Selection"(u16 0 ("milliseconds to wait")) -> ()
